vi "RDG822 User.vi"() -> ()   [LabVIEW 2021]
panel:
  in  "MenuCont":u32=1
  in  "RemoveReq?":bool=TRUE
  in  "userID":string="0001"
  out "error out":errorcluster
  in  "E:\\Study\\НИР_Маг\\FP":path=path "E:/Study/НИР_Маг/FP"
  in  "error in":errorcluster
  in  "DutyDBL":dbl=50.0 format="%.3f"
  out "DutyStr":string="50.000 %"
  in  "Noise":bool
  in  "Pulse":bool
  in  "Ramp":bool
  in  "Square":bool
  in  "Sine":bool
  in  "Slider":bool
  in  "PhaseDBL":dbl format="%.3f"
  in  "OK":bool
  out "PhaseStr":string="0.000 °"
  in  "LowL":dbl=-2.5 format="%.4f"
  in  "Offset":dbl format="%.4f"
  out "Offset-LowL":string="0.0000 Vdc"
  in  "Offset/LowL":bool
  in  "HighL":dbl=1.0 format="%.4f"
  in  "Ampl":dbl=5.0 format="%.4f"
  out "Ampl-HighL":string="5.0000 Vpp"
  in  "Ampl/HighL":bool
  in  "Freq":dbl=1.0 format="%.6f"
  in  "Period":dbl=1.0 format="%.7f"
  out "Freq-Period":string="1000.000000000 kHz"
  in  "Freq/Period":bool
  in  "Left":bool
  in  "Right":bool
  in  "Out2":bool
  in  "Out1":bool
  out "Screen":picture
  in  "Menu":bool
  in  "Home":bool
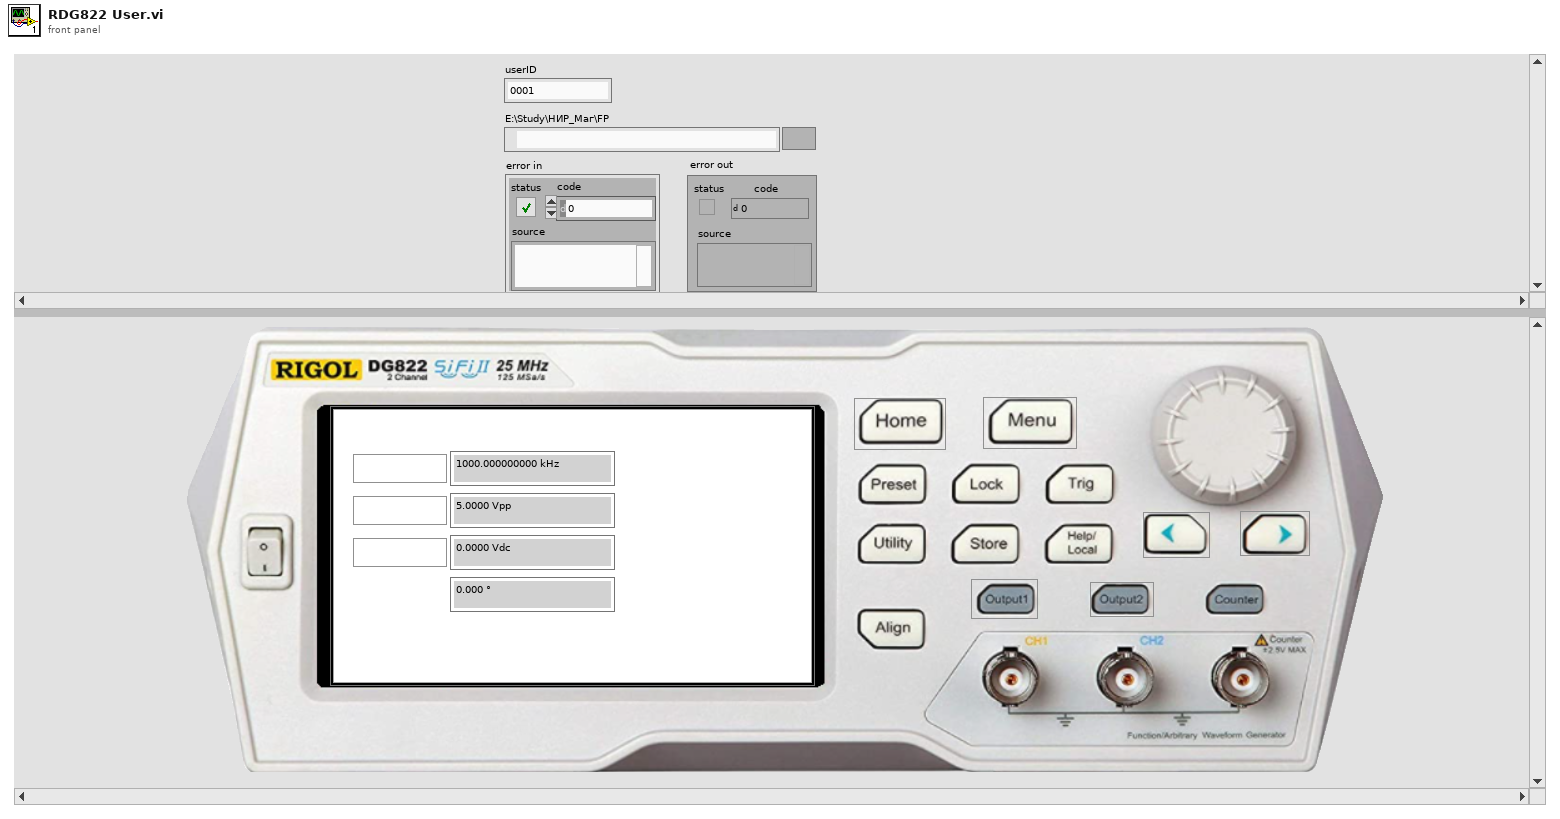
[diagram p1: front panel]
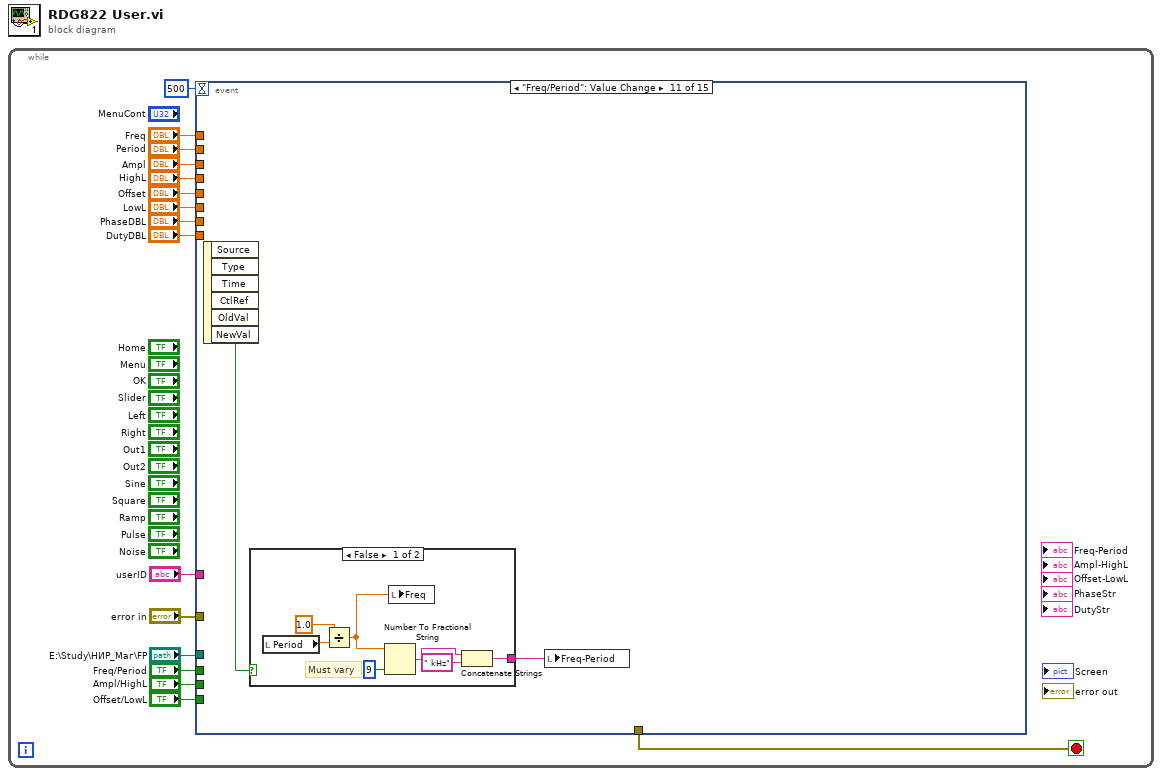
[diagram p0: block diagram]
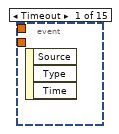
[diagram p2: hidden frame]
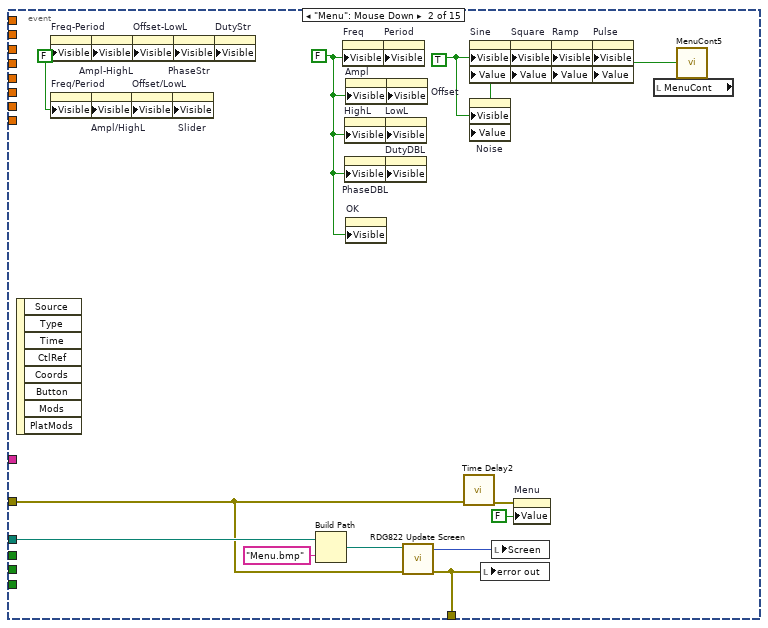
[diagram p3: hidden frame]
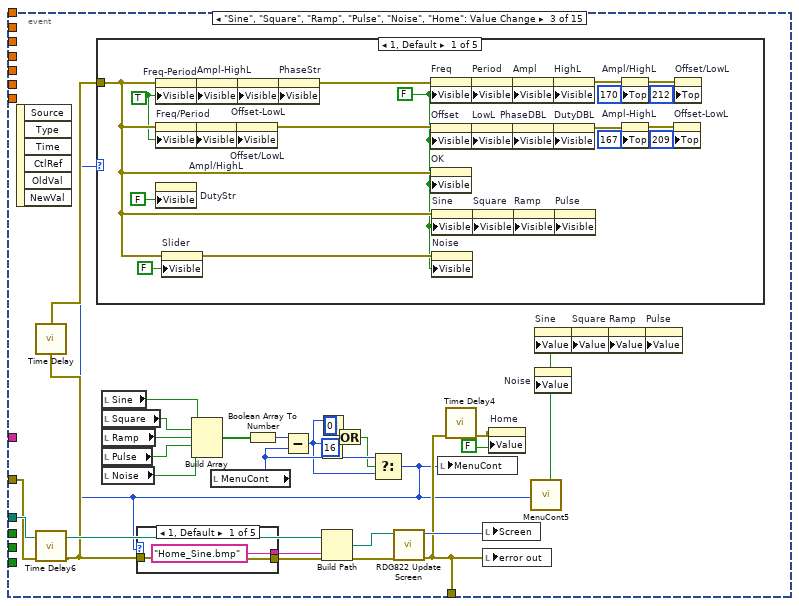
[diagram p4: hidden frame]
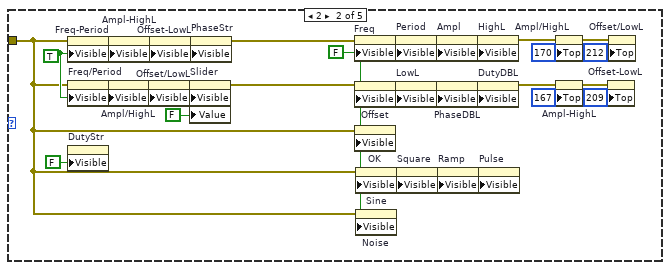
[diagram p5: hidden frame]
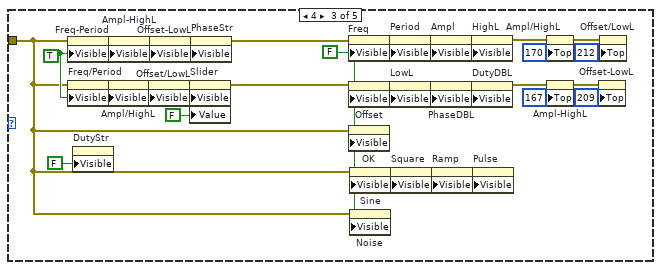
[diagram p6: hidden frame]
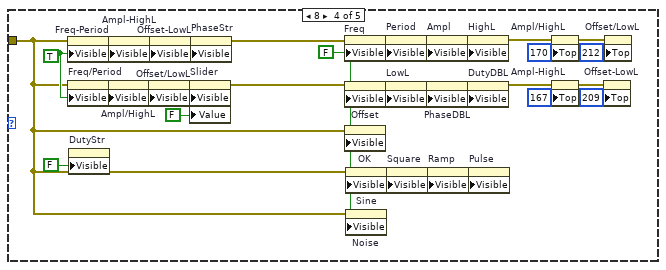
[diagram p7: hidden frame]
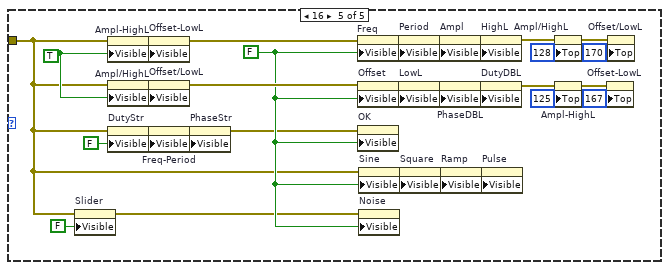
[diagram p8: hidden frame]
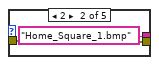
[diagram p9: hidden frame]
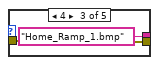
[diagram p10: hidden frame]
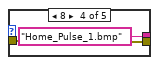
[diagram p11: hidden frame]
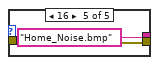
[diagram p12: hidden frame]
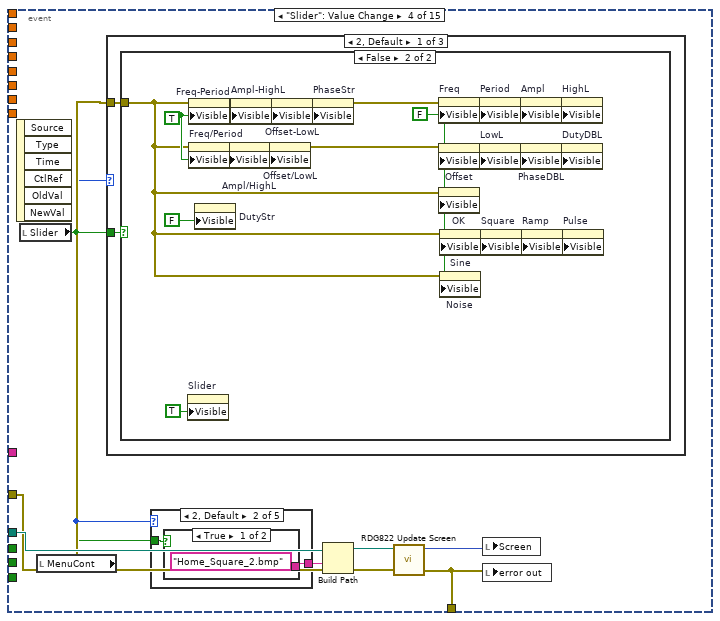
[diagram p13: hidden frame]
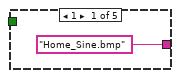
[diagram p14: hidden frame]
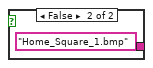
[diagram p15: hidden frame]
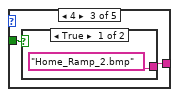
[diagram p16: hidden frame]
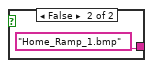
[diagram p17: hidden frame]
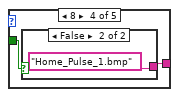
[diagram p18: hidden frame]
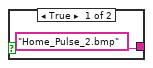
[diagram p19: hidden frame]
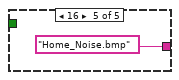
[diagram p20: hidden frame]
diagram:
  n1 = while {
    stop <- w16 stop-if-true
    n2 = event shown="[10] \"Freq/Period\": Value Change" {
      selector: _ -> [_ _ _ _ _ _ _ _ _ _ _ _ _ _ _]
      dyn-events: _ -> [_ _ _ _ _ _ _ _ _ _ _ _ _ _ _]
      timeout: 500 -> [_ _ _ _ _ _ _ _ _ _ _ _ _ _ _]
      tunnel: [_ w39 w64 w236 w393 w770 w803 w836 w868 w889 _ _ _ w1009 _] -> w16
      tunnel: "error in" -> [_ w37 w52 w235 w384 _ _ _ _ _ _ _ _ w1027 _]
      tunnel: "E:\\Study\\НИР_Маг\\FP" -> [_ w40 w68 w237 w397 w785 w818 w851 w874 w895 _ _ _ w1015 _]
      tunnel: "Freq/Period" -> [_ _ _ _ w400 w783 _ _ _ _ _ _ _ w1044 _]
      tunnel: "Ampl/HighL" -> [_ _ _ _ w399 _ w813 _ _ _ _ _ _ w1045 _]
      tunnel: "Freq" -> [_ _ _ _ _ _ _ _ _ _ _ _ _ w1043 _]
      tunnel: "Ampl" -> [_ _ _ _ _ _ _ _ _ _ _ _ _ w1041 _]
      tunnel: "Period" -> [_ _ _ _ _ _ _ _ _ _ _ _ _ w1042 _]
      tunnel: "HighL" -> [_ _ _ _ _ _ _ _ _ _ _ _ _ w1038 _]
      tunnel: "Offset/LowL" -> [_ _ _ _ w398 _ _ w841 _ _ _ _ _ w1040 _]
      tunnel: "Offset" -> [_ _ _ _ _ _ _ _ _ _ _ _ _ w1004 _]
      tunnel: "LowL" -> [_ _ _ _ _ _ _ _ _ _ _ _ _ w1039 _]
      tunnel: "PhaseDBL" -> [_ _ _ _ _ _ _ _ _ _ _ _ _ w1032 _]
      tunnel: "userID" -> [_ _ _ _ _ _ _ _ _ _ _ _ _ w1026 _]
      tunnel: "DutyDBL" -> [_ _ _ _ _ _ _ _ _ _ _ _ _ w1001 _]
      event Timeout {
        n3 = event-data() -> ()  [unwired: 1 in, 3 out]
      }
      event "Menu": Mouse Down {
        w25 = TRUE ("Visible")
        w18 = FALSE ("Visible")
        w17 = FALSE ("Visible")
        n4 = event-data() -> ()  [unwired: 1 in, 8 out]
        n5 = property on="Freq-Period" class="Str"("Visible"=w18) -> (error out=w36:errorcluster)  [unwired: 2 in, 1 out]
        n6 = property on="Freq/Period" class="Bool (strict)"("Visible"=w18) -> (error out=w33:errorcluster)  [unwired: 2 in, 1 out]
        n7 = property on="Ampl/HighL" class="Bool (strict)"(error in=w33, "Visible"=w18) -> (error out=w32:errorcluster)  [unwired: 1 in, 1 out]
        n8 = property on="Ampl-HighL" class="Str"(error in=w36, "Visible"=w18) -> (error out=w35:errorcluster)  [unwired: 1 in, 1 out]
        n9 = property on="Offset/LowL" class="Bool (strict)"(error in=w32, "Visible"=w18) -> (error out=w29:errorcluster)  [unwired: 1 in, 1 out]
        n10 = property on="Offset-LowL" class="Str"(error in=w35, "Visible"=w18) -> (error out=w34:errorcluster)  [unwired: 1 in, 1 out]
        n11 = property on="Slider" class="Bool (strict)"(error in=w29, "Visible"=w18) -> ()  [unwired: 1 in, 2 out]
        n12 = property on="PhaseStr" class="Str"(error in=w34, "Visible"=w18) -> ()  [unwired: 1 in, 2 out]
        n13 = property on="DutyStr" class="Str"("Visible"=w18) -> ()  [unwired: 2 in, 2 out]
        n14 = Build Path(base path=w40, name or relative path="Menu.bmp") -> (appended path=w41:path)
        n15 = property on="Freq" class="DigNum (strict)"("Visible"=w17) -> (error out=w31:errorcluster)  [unwired: 2 in, 1 out]
        n16 = property on="HighL" class="DigNum (strict)"("Visible"=w17) -> ()  [unwired: 2 in, 2 out]
        n17 = property on="PhaseDBL" class="DigNum (strict)"("Visible"=w17) -> ()  [unwired: 2 in, 2 out]
        n18 = property on="Ampl" class="DigNum (strict)"("Visible"=w17) -> (error out=w30:errorcluster)  [unwired: 2 in, 1 out]
        n19 = property on="OK" class="Bool (strict)"("Visible"=w17) -> ()  [unwired: 2 in, 2 out]
        n20 = property on="Period" class="DigNum (strict)"(error in=w31, "Visible"=w17) -> ()  [unwired: 1 in, 2 out]
        n21 = property on="LowL" class="DigNum (strict)"("Visible"=w17) -> ()  [unwired: 2 in, 2 out]
        n22 = property on="DutyDBL" class="DigNum (strict)"("Visible"=w17) -> ()  [unwired: 2 in, 2 out]
        n23 = property on="Offset" class="DigNum (strict)"(error in=w30, "Visible"=w17) -> ()  [unwired: 1 in, 2 out]
        n24 = call "RDG822 Update Screen.vi"("error in"=w37, "Path to file"=w41) -> ("error out"=w39:errorcluster, "Screen"=w38:picture)  [unwired: 8 in]
        n25 = call "Time Delay2"("error in (no error)"=w37) -> ("error out"=w44:errorcluster)  [unwired: 10 in]
        n26 = local write "error out"(w39) -> ()
        n27 = local write "Screen"(w38) -> ()
        n28 = property on="Menu" class="Bool (strict)"(error in=w44, "Value"=FALSE ("Visible")) -> ()  [unwired: 1 in, 2 out]
        n29 = local read "MenuCont"() -> (w24:u32)
        n30 = call "MenuCont5.vi"("MenuID"=w24) -> ("Sine"=w23:bool, "Square"=w22:bool, "Ramp"=w21:bool, "Pulse"=w20:bool, "Noise"=w19:bool)  [unwired: 10 in]
        n31 = property on="Sine" class="Bool (strict)"("Visible"=w25, "Value"=w23) -> (error out=w28:errorcluster)  [unwired: 2 in, 1 out]
        n32 = property on="Noise" class="Bool (strict)"("Visible"=w25, "Value"=w19) -> ()  [unwired: 2 in, 2 out]
        n33 = property on="Square" class="Bool (strict)"(error in=w28, "Visible"=w25, "Value"=w22) -> (error out=w27:errorcluster)  [unwired: 1 in, 1 out]
        n34 = property on="Ramp" class="Bool (strict)"(error in=w27, "Visible"=w25, "Value"=w21) -> (error out=w26:errorcluster)  [unwired: 1 in, 1 out]
        n35 = property on="Pulse" class="Bool (strict)"(error in=w26, "Visible"=w25, "Value"=w20) -> ()  [unwired: 1 in, 2 out]
      }
      event "Sine", "Square", "Ramp", "Pulse", "Noise", "Home": Value Change {
        n36 = event-data() -> ()  [unwired: 1 in, 6 out]
        n37 = call "Time Delay6"("error in (no error)"=w52) -> ("error out"=w49:errorcluster)  [unwired: 10 in]
        n38 = call "Time Delay"("error in (no error)"=w49) -> ("error out"=w50:errorcluster)  [unwired: 10 in]
        n39 = local read "Sine"() -> (w73:bool)
        n40 = local read "Square"() -> (w74:bool)
        n41 = local read "Ramp"() -> (w75:bool)
        n42 = local read "Pulse"() -> (w72:bool)
        n43 = local read "Noise"() -> (w71:bool)
        n44 = Build Array(w73, w74, w75, w72, w71) -> (w76:bool[])
        n45 = local read "MenuCont"() -> (w48:u32)
        n46 = Boolean Array To Number(Boolean array=w76) -> (number=w70:u32)
        n47 = Subtract(x=w70, y=w48) -> (x-y=w47:u32)
        n48 = Greater?(x=w47, y=u32 16) -> (0:w54:bool)
        n49 = Less Or Equal?(x=w47, y=u32 0) -> (x <= y?=w55:bool)
        n50 = Or(x=w55, y=w54) -> (x .or. y?=w46:bool)
        n51 = Select(t=w48, s=w46, f=w47) -> (s? t:f=w45:u32)
        n52 = case shown="1, Default" w45 {
          tunnel: w50 -> [w91 w119 w148 w177 w195]
          frame 1, Default {
            w80 = TRUE ("Visible")
            w81 = FALSE ("Visible")
            n53 = property on="Freq-Period" class="Str"(error in=w91, "Visible"=w80) -> (error out=w107:errorcluster)  [unwired: 1 in, 1 out]
            n54 = property on="Freq/Period" class="Bool (strict)"(error in=w91, "Visible"=w80) -> (error out=w104:errorcluster)  [unwired: 1 in, 1 out]
            n55 = property on="DutyStr" class="Str"("Visible"=FALSE) -> ()  [unwired: 2 in, 2 out]
            n56 = property on="Slider" class="Bool (strict)"(error in=w91, "Visible"=FALSE) -> (error out=w92:errorcluster)  [unwired: 1 in, 1 out]
            n57 = property on="Ampl/HighL" class="Bool (strict)"(error in=w104, "Visible"=w80) -> (error out=w103:errorcluster)  [unwired: 1 in, 1 out]
            n58 = property on="Ampl-HighL" class="Str"(error in=w107, "Visible"=w80) -> (error out=w106:errorcluster)  [unwired: 1 in, 1 out]
            n59 = property on="Offset/LowL" class="Bool (strict)"(error in=w103, "Visible"=w80) -> (error out=w93:errorcluster)  [unwired: 1 in, 1 out]
            n60 = property on="Offset-LowL" class="Str"(error in=w106, "Visible"=w80) -> (error out=w105:errorcluster)  [unwired: 1 in, 1 out]
            n61 = property on="PhaseStr" class="Str"(error in=w105, "Visible"=w80) -> (error out=w98:errorcluster)  [unwired: 1 in, 1 out]
            n62 = property on="Freq" class="DigNum (strict)"(error in=w98, "Visible"=w81) -> (error out=w97:errorcluster)  [unwired: 1 in, 1 out]
            n63 = property on="Offset" class="DigNum (strict)"(error in=w93, "Visible"=w81) -> (error out=w94:errorcluster)  [unwired: 1 in, 1 out]
            n64 = property on="OK" class="Bool (strict)"(error in=w91, "Visible"=w81) -> ()  [unwired: 1 in, 2 out]
            n65 = property on="Sine" class="Bool (strict)"(error in=w91, "Visible"=w81) -> (error out=w101:errorcluster)  [unwired: 1 in, 1 out]
            n66 = property on="Noise" class="Bool (strict)"(error in=w92, "Visible"=w81) -> ()  [unwired: 1 in, 2 out]
            n67 = property on="Period" class="DigNum (strict)"(error in=w97, "Visible"=w81) -> (error out=w96:errorcluster)  [unwired: 1 in, 1 out]
            n68 = property on="LowL" class="DigNum (strict)"(error in=w94, "Visible"=w81) -> (error out=w95:errorcluster)  [unwired: 1 in, 1 out]
            n69 = property on="Square" class="Bool (strict)"(error in=w101, "Visible"=w81) -> (error out=w100:errorcluster)  [unwired: 1 in, 1 out]
            n70 = property on="Ampl" class="DigNum (strict)"(error in=w96, "Visible"=w81) -> (error out=w102:errorcluster)  [unwired: 1 in, 1 out]
            n71 = property on="PhaseDBL" class="DigNum (strict)"(error in=w95, "Visible"=w81) -> (error out=w82:errorcluster)  [unwired: 1 in, 1 out]
            n72 = property on="Ramp" class="Bool (strict)"(error in=w100, "Visible"=w81) -> (error out=w99:errorcluster)  [unwired: 1 in, 1 out]
            n73 = property on="HighL" class="DigNum (strict)"(error in=w102, "Visible"=w81) -> (error out=w88:errorcluster)  [unwired: 1 in, 1 out]
            n74 = property on="DutyDBL" class="DigNum (strict)"("Visible"=w81) -> ()  [unwired: 2 in, 2 out]
            n75 = property on="Pulse" class="Bool (strict)"(error in=w99, "Visible"=w81) -> ()  [unwired: 1 in, 2 out]
            n76 = property on="Ampl/HighL" class="Bool (strict)"(error in=w88, "Top"=170 ("Position:Top")) -> (error out=w86:errorcluster)  [unwired: 1 in, 1 out]
            n77 = property on="Ampl-HighL" class="Str"(error in=w82, "Top"=167 ("Position:Top")) -> (error out=w83:errorcluster)  [unwired: 1 in, 1 out]
            n78 = property on="Offset-LowL" class="Str"(error in=w83, "Top"=209 ("Position:Top")) -> ()  [unwired: 1 in, 2 out]
            n79 = property on="Offset/LowL" class="Bool (strict)"(error in=w86, "Top"=212 ("Position:Top")) -> ()  [unwired: 1 in, 2 out]
          }
          frame 2 {
            w129 = TRUE ("Visible")
            w109 = FALSE ("Visible")
            n80 = property on="Freq-Period" class="Str"(error in=w119, "Visible"=w129) -> (error out=w136:errorcluster)  [unwired: 1 in, 1 out]
            n81 = property on="Freq/Period" class="Bool (strict)"(error in=w119, "Visible"=w129) -> (error out=w133:errorcluster)  [unwired: 1 in, 1 out]
            n82 = property on="DutyStr" class="Str"("Visible"=FALSE) -> ()  [unwired: 2 in, 2 out]
            n83 = property on="Ampl/HighL" class="Bool (strict)"(error in=w133, "Visible"=w129) -> (error out=w132:errorcluster)  [unwired: 1 in, 1 out]
            n84 = property on="Ampl-HighL" class="Str"(error in=w136, "Visible"=w129) -> (error out=w135:errorcluster)  [unwired: 1 in, 1 out]
            n85 = property on="Offset/LowL" class="Bool (strict)"(error in=w132, "Visible"=w129) -> (error out=w130:errorcluster)  [unwired: 1 in, 1 out]
            n86 = property on="Offset-LowL" class="Str"(error in=w135, "Visible"=w129) -> (error out=w134:errorcluster)  [unwired: 1 in, 1 out]
            n87 = property on="Slider" class="Bool (strict)"(error in=w130, "Visible"=w129, "Value"=FALSE ("Slider")) -> (error out=w124:errorcluster)  [unwired: 1 in, 1 out]
            n88 = property on="PhaseStr" class="Str"(error in=w134, "Visible"=w129) -> (error out=w125:errorcluster)  [unwired: 1 in, 1 out]
            n89 = property on="Freq" class="DigNum (strict)"(error in=w125, "Visible"=w109) -> (error out=w123:errorcluster)  [unwired: 1 in, 1 out]
            n90 = property on="Offset" class="DigNum (strict)"(error in=w124, "Visible"=w109) -> (error out=w120:errorcluster)  [unwired: 1 in, 1 out]
            n91 = property on="OK" class="Bool (strict)"(error in=w119, "Visible"=w109) -> ()  [unwired: 1 in, 2 out]
            n92 = property on="Sine" class="Bool (strict)"(error in=w119, "Visible"=w109) -> (error out=w128:errorcluster)  [unwired: 1 in, 1 out]
            n93 = property on="Noise" class="Bool (strict)"(error in=w119, "Visible"=w109) -> ()  [unwired: 1 in, 2 out]
            n94 = property on="Period" class="DigNum (strict)"(error in=w123, "Visible"=w109) -> (error out=w122:errorcluster)  [unwired: 1 in, 1 out]
            n95 = property on="LowL" class="DigNum (strict)"(error in=w120, "Visible"=w109) -> (error out=w121:errorcluster)  [unwired: 1 in, 1 out]
            n96 = property on="Square" class="Bool (strict)"(error in=w128, "Visible"=w109) -> (error out=w127:errorcluster)  [unwired: 1 in, 1 out]
            n97 = property on="Ampl" class="DigNum (strict)"(error in=w122, "Visible"=w109) -> (error out=w131:errorcluster)  [unwired: 1 in, 1 out]
            n98 = property on="PhaseDBL" class="DigNum (strict)"(error in=w121, "Visible"=w109) -> (error out=w111:errorcluster)  [unwired: 1 in, 1 out]
            n99 = property on="Ramp" class="Bool (strict)"(error in=w127, "Visible"=w109) -> (error out=w126:errorcluster)  [unwired: 1 in, 1 out]
            n100 = property on="HighL" class="DigNum (strict)"(error in=w131, "Visible"=w109) -> (error out=w110:errorcluster)  [unwired: 1 in, 1 out]
            n101 = property on="DutyDBL" class="DigNum (strict)"("Visible"=w109) -> ()  [unwired: 2 in, 2 out]
            n102 = property on="Pulse" class="Bool (strict)"(error in=w126, "Visible"=w109) -> ()  [unwired: 1 in, 2 out]
            n103 = property on="Ampl/HighL" class="Bool (strict)"(error in=w110, "Top"=170 ("Position:Top")) -> (error out=w115:errorcluster)  [unwired: 1 in, 1 out]
            n104 = property on="Ampl-HighL" class="Str"(error in=w111, "Top"=167 ("Position:Top")) -> (error out=w112:errorcluster)  [unwired: 1 in, 1 out]
            n105 = property on="Offset-LowL" class="Str"(error in=w112, "Top"=209 ("Position:Top")) -> ()  [unwired: 1 in, 2 out]
            n106 = property on="Offset/LowL" class="Bool (strict)"(error in=w115, "Top"=212 ("Position:Top")) -> ()  [unwired: 1 in, 2 out]
          }
          frame 4 {
            w158 = TRUE ("Visible")
            w138 = FALSE ("Visible")
            n107 = property on="Freq-Period" class="Str"(error in=w148, "Visible"=w158) -> (error out=w165:errorcluster)  [unwired: 1 in, 1 out]
            n108 = property on="Freq/Period" class="Bool (strict)"(error in=w148, "Visible"=w158) -> (error out=w162:errorcluster)  [unwired: 1 in, 1 out]
            n109 = property on="DutyStr" class="Str"("Visible"=FALSE) -> ()  [unwired: 2 in, 2 out]
            n110 = property on="Ampl/HighL" class="Bool (strict)"(error in=w162, "Visible"=w158) -> (error out=w161:errorcluster)  [unwired: 1 in, 1 out]
            n111 = property on="Ampl-HighL" class="Str"(error in=w165, "Visible"=w158) -> (error out=w164:errorcluster)  [unwired: 1 in, 1 out]
            n112 = property on="Offset/LowL" class="Bool (strict)"(error in=w161, "Visible"=w158) -> (error out=w159:errorcluster)  [unwired: 1 in, 1 out]
            n113 = property on="Offset-LowL" class="Str"(error in=w164, "Visible"=w158) -> (error out=w163:errorcluster)  [unwired: 1 in, 1 out]
            n114 = property on="Slider" class="Bool (strict)"(error in=w159, "Visible"=w158, "Value"=FALSE ("Slider")) -> (error out=w153:errorcluster)  [unwired: 1 in, 1 out]
            n115 = property on="PhaseStr" class="Str"(error in=w163, "Visible"=w158) -> (error out=w154:errorcluster)  [unwired: 1 in, 1 out]
            n116 = property on="Freq" class="DigNum (strict)"(error in=w154, "Visible"=w138) -> (error out=w152:errorcluster)  [unwired: 1 in, 1 out]
            n117 = property on="Offset" class="DigNum (strict)"(error in=w153, "Visible"=w138) -> (error out=w149:errorcluster)  [unwired: 1 in, 1 out]
            n118 = property on="OK" class="Bool (strict)"(error in=w148, "Visible"=w138) -> ()  [unwired: 1 in, 2 out]
            n119 = property on="Sine" class="Bool (strict)"(error in=w148, "Visible"=w138) -> (error out=w157:errorcluster)  [unwired: 1 in, 1 out]
            n120 = property on="Noise" class="Bool (strict)"(error in=w148, "Visible"=w138) -> ()  [unwired: 1 in, 2 out]
            n121 = property on="Period" class="DigNum (strict)"(error in=w152, "Visible"=w138) -> (error out=w151:errorcluster)  [unwired: 1 in, 1 out]
            n122 = property on="LowL" class="DigNum (strict)"(error in=w149, "Visible"=w138) -> (error out=w150:errorcluster)  [unwired: 1 in, 1 out]
            n123 = property on="Square" class="Bool (strict)"(error in=w157, "Visible"=w138) -> (error out=w156:errorcluster)  [unwired: 1 in, 1 out]
            n124 = property on="Ampl" class="DigNum (strict)"(error in=w151, "Visible"=w138) -> (error out=w160:errorcluster)  [unwired: 1 in, 1 out]
            n125 = property on="PhaseDBL" class="DigNum (strict)"(error in=w150, "Visible"=w138) -> (error out=w139:errorcluster)  [unwired: 1 in, 1 out]
            n126 = property on="Ramp" class="Bool (strict)"(error in=w156, "Visible"=w138) -> (error out=w155:errorcluster)  [unwired: 1 in, 1 out]
            n127 = property on="HighL" class="DigNum (strict)"(error in=w160, "Visible"=w138) -> (error out=w140:errorcluster)  [unwired: 1 in, 1 out]
            n128 = property on="DutyDBL" class="DigNum (strict)"("Visible"=w138) -> ()  [unwired: 2 in, 2 out]
            n129 = property on="Pulse" class="Bool (strict)"(error in=w155, "Visible"=w138) -> ()  [unwired: 1 in, 2 out]
            n130 = property on="Ampl/HighL" class="Bool (strict)"(error in=w140, "Top"=170 ("Position:Top")) -> (error out=w144:errorcluster)  [unwired: 1 in, 1 out]
            n131 = property on="Ampl-HighL" class="Str"(error in=w139, "Top"=167 ("Position:Top")) -> (error out=w141:errorcluster)  [unwired: 1 in, 1 out]
            n132 = property on="Offset-LowL" class="Str"(error in=w141, "Top"=209 ("Position:Top")) -> ()  [unwired: 1 in, 2 out]
            n133 = property on="Offset/LowL" class="Bool (strict)"(error in=w144, "Top"=212 ("Position:Top")) -> ()  [unwired: 1 in, 2 out]
          }
          frame 8 {
            w187 = TRUE ("Visible")
            w167 = FALSE ("Visible")
            n134 = property on="Freq-Period" class="Str"(error in=w177, "Visible"=w187) -> (error out=w194:errorcluster)  [unwired: 1 in, 1 out]
            n135 = property on="Freq/Period" class="Bool (strict)"(error in=w177, "Visible"=w187) -> (error out=w191:errorcluster)  [unwired: 1 in, 1 out]
            n136 = property on="DutyStr" class="Str"("Visible"=FALSE) -> ()  [unwired: 2 in, 2 out]
            n137 = property on="Ampl/HighL" class="Bool (strict)"(error in=w191, "Visible"=w187) -> (error out=w190:errorcluster)  [unwired: 1 in, 1 out]
            n138 = property on="Ampl-HighL" class="Str"(error in=w194, "Visible"=w187) -> (error out=w193:errorcluster)  [unwired: 1 in, 1 out]
            n139 = property on="Offset/LowL" class="Bool (strict)"(error in=w190, "Visible"=w187) -> (error out=w188:errorcluster)  [unwired: 1 in, 1 out]
            n140 = property on="Offset-LowL" class="Str"(error in=w193, "Visible"=w187) -> (error out=w192:errorcluster)  [unwired: 1 in, 1 out]
            n141 = property on="Slider" class="Bool (strict)"(error in=w188, "Visible"=w187, "Value"=FALSE ("Slider")) -> (error out=w182:errorcluster)  [unwired: 1 in, 1 out]
            n142 = property on="PhaseStr" class="Str"(error in=w192, "Visible"=w187) -> (error out=w183:errorcluster)  [unwired: 1 in, 1 out]
            n143 = property on="Freq" class="DigNum (strict)"(error in=w183, "Visible"=w167) -> (error out=w181:errorcluster)  [unwired: 1 in, 1 out]
            n144 = property on="Offset" class="DigNum (strict)"(error in=w182, "Visible"=w167) -> (error out=w178:errorcluster)  [unwired: 1 in, 1 out]
            n145 = property on="OK" class="Bool (strict)"(error in=w177, "Visible"=w167) -> ()  [unwired: 1 in, 2 out]
            n146 = property on="Sine" class="Bool (strict)"(error in=w177, "Visible"=w167) -> (error out=w186:errorcluster)  [unwired: 1 in, 1 out]
            n147 = property on="Noise" class="Bool (strict)"(error in=w177, "Visible"=w167) -> ()  [unwired: 1 in, 2 out]
            n148 = property on="Period" class="DigNum (strict)"(error in=w181, "Visible"=w167) -> (error out=w180:errorcluster)  [unwired: 1 in, 1 out]
            n149 = property on="LowL" class="DigNum (strict)"(error in=w178, "Visible"=w167) -> (error out=w179:errorcluster)  [unwired: 1 in, 1 out]
            n150 = property on="Square" class="Bool (strict)"(error in=w186, "Visible"=w167) -> (error out=w185:errorcluster)  [unwired: 1 in, 1 out]
            n151 = property on="Ampl" class="DigNum (strict)"(error in=w180, "Visible"=w167) -> (error out=w189:errorcluster)  [unwired: 1 in, 1 out]
            n152 = property on="PhaseDBL" class="DigNum (strict)"(error in=w179, "Visible"=w167) -> (error out=w168:errorcluster)  [unwired: 1 in, 1 out]
            n153 = property on="Ramp" class="Bool (strict)"(error in=w185, "Visible"=w167) -> (error out=w184:errorcluster)  [unwired: 1 in, 1 out]
            n154 = property on="HighL" class="DigNum (strict)"(error in=w189, "Visible"=w167) -> (error out=w169:errorcluster)  [unwired: 1 in, 1 out]
            n155 = property on="DutyDBL" class="DigNum (strict)"("Visible"=w167) -> ()  [unwired: 2 in, 2 out]
            n156 = property on="Pulse" class="Bool (strict)"(error in=w184, "Visible"=w167) -> ()  [unwired: 1 in, 2 out]
            n157 = property on="Ampl/HighL" class="Bool (strict)"(error in=w169, "Top"=170 ("Position:Top")) -> (error out=w173:errorcluster)  [unwired: 1 in, 1 out]
            n158 = property on="Ampl-HighL" class="Str"(error in=w168, "Top"=167 ("Position:Top")) -> (error out=w170:errorcluster)  [unwired: 1 in, 1 out]
            n159 = property on="Offset-LowL" class="Str"(error in=w170, "Top"=209 ("Position:Top")) -> ()  [unwired: 1 in, 2 out]
            n160 = property on="Offset/LowL" class="Bool (strict)"(error in=w173, "Top"=212 ("Position:Top")) -> ()  [unwired: 1 in, 2 out]
          }
          frame 16 {
            w198 = FALSE ("Visible")
            w218 = TRUE ("Visible")
            w199 = FALSE ("Visible")
            n161 = property on="Slider" class="Bool (strict)"(error in=w195, "Visible"=FALSE) -> ()  [unwired: 1 in, 2 out]
            n162 = property on="Ampl-HighL" class="Str"(error in=w195, "Visible"=w218) -> (error out=w221:errorcluster)  [unwired: 1 in, 1 out]
            n163 = property on="Ampl/HighL" class="Bool (strict)"(error in=w195, "Visible"=w218) -> (error out=w220:errorcluster)  [unwired: 1 in, 1 out]
            n164 = property on="DutyStr" class="Str"(error in=w195, "Visible"=w198) -> (error out=w197:errorcluster)  [unwired: 1 in, 1 out]
            n165 = property on="Offset-LowL" class="Str"(error in=w221, "Visible"=w218) -> (error out=w208:errorcluster)  [unwired: 1 in, 1 out]
            n166 = property on="Offset/LowL" class="Bool (strict)"(error in=w220, "Visible"=w218) -> (error out=w210:errorcluster)  [unwired: 1 in, 1 out]
            n167 = property on="Freq-Period" class="Str"(error in=w197, "Visible"=w198) -> (error out=w196:errorcluster)  [unwired: 1 in, 1 out]
            n168 = property on="PhaseStr" class="Str"(error in=w196, "Visible"=w198) -> ()  [unwired: 1 in, 2 out]
            n169 = property on="Freq" class="DigNum (strict)"(error in=w208, "Visible"=w199) -> (error out=w214:errorcluster)  [unwired: 1 in, 1 out]
            n170 = property on="Offset" class="DigNum (strict)"(error in=w210, "Visible"=w199) -> (error out=w211:errorcluster)  [unwired: 1 in, 1 out]
            n171 = property on="OK" class="Bool (strict)"(error in=w195, "Visible"=w199) -> ()  [unwired: 1 in, 2 out]
            n172 = property on="Sine" class="Bool (strict)"(error in=w195, "Visible"=w199) -> (error out=w217:errorcluster)  [unwired: 1 in, 1 out]
            n173 = property on="Noise" class="Bool (strict)"(error in=w195, "Visible"=w199) -> ()  [unwired: 1 in, 2 out]
            n174 = property on="Period" class="DigNum (strict)"(error in=w214, "Visible"=w199) -> (error out=w213:errorcluster)  [unwired: 1 in, 1 out]
            n175 = property on="LowL" class="DigNum (strict)"(error in=w211, "Visible"=w199) -> (error out=w212:errorcluster)  [unwired: 1 in, 1 out]
            n176 = property on="Square" class="Bool (strict)"(error in=w217, "Visible"=w199) -> (error out=w216:errorcluster)  [unwired: 1 in, 1 out]
            n177 = property on="Ampl" class="DigNum (strict)"(error in=w213, "Visible"=w199) -> (error out=w219:errorcluster)  [unwired: 1 in, 1 out]
            n178 = property on="PhaseDBL" class="DigNum (strict)"(error in=w212, "Visible"=w199) -> (error out=w200:errorcluster)  [unwired: 1 in, 1 out]
            n179 = property on="Ramp" class="Bool (strict)"(error in=w216, "Visible"=w199) -> (error out=w215:errorcluster)  [unwired: 1 in, 1 out]
            n180 = property on="HighL" class="DigNum (strict)"(error in=w219, "Visible"=w199) -> (error out=w201:errorcluster)  [unwired: 1 in, 1 out]
            n181 = property on="DutyDBL" class="DigNum (strict)"("Visible"=w199) -> ()  [unwired: 2 in, 2 out]
            n182 = property on="Pulse" class="Bool (strict)"(error in=w215, "Visible"=w199) -> ()  [unwired: 1 in, 2 out]
            n183 = property on="Ampl/HighL" class="Bool (strict)"(error in=w201, "Top"=128 ("Position:Top")) -> (error out=w205:errorcluster)  [unwired: 1 in, 1 out]
            n184 = property on="Ampl-HighL" class="Str"(error in=w200, "Top"=125 ("Position:Top")) -> (error out=w202:errorcluster)  [unwired: 1 in, 1 out]
            n185 = property on="Offset-LowL" class="Str"(error in=w202, "Top"=167 ("Position:Top")) -> ()  [unwired: 1 in, 2 out]
            n186 = property on="Offset/LowL" class="Bool (strict)"(error in=w205, "Top"=170 ("Position:Top")) -> ()  [unwired: 1 in, 2 out]
          }
        }
        n187 = case shown="1, Default" w45 {
          tunnel: ["Home_Sine.bmp" "Home_Square_1.bmp" "Home_Ramp_1.bmp" "Home_Pulse_1.bmp" "Home_Noise.bmp"] -> w69
          tunnel: w49 -> [w222 w224 w226 w228 w230]
          tunnel: [w222 w224 w226 w228 w230] -> w51
          frame 1, Default {
          }
          frame 2 {
          }
          frame 4 {
          }
          frame 8 {
          }
          frame 16 {
          }
        }
        n188 = Build Path(base path=w68, name or relative path=w69) -> (appended path=w78:path)
        n189 = call "RDG822 Update Screen.vi"("error in"=w51, "Path to file"=w78) -> ("error out"=w64:errorcluster, "Screen"=w77:picture)  [unwired: 8 in]
        n190 = local write "MenuCont"(w45) -> ()
        n191 = call "Time Delay4"("error in (no error)"=w64) -> ("error out"=w66:errorcluster)  [unwired: 10 in]
        n192 = local write "Screen"(w77) -> ()
        n193 = local write "error out"(w64) -> ()
        n194 = property on="Home" class="Bool (strict)"(error in=w66, "Value"=FALSE ("Home")) -> ()  [unwired: 1 in, 2 out]
        n195 = call "MenuCont5.vi"("MenuID"=w45) -> ("Sine"=w60:bool, "Square"=w59:bool, "Ramp"=w58:bool, "Pulse"=w57:bool, "Noise"=w56:bool)  [unwired: 10 in]
        n196 = property on="Sine" class="Bool (strict)"("Value"=w60) -> (error out=w63:errorcluster)  [unwired: 2 in, 1 out]
        n197 = property on="Noise" class="Bool (strict)"("Value"=w56) -> ()  [unwired: 2 in, 2 out]
        n198 = property on="Square" class="Bool (strict)"(error in=w63, "Value"=w59) -> (error out=w62:errorcluster)  [unwired: 1 in, 1 out]
        n199 = property on="Ramp" class="Bool (strict)"(error in=w62, "Value"=w58) -> (error out=w61:errorcluster)  [unwired: 1 in, 1 out]
        n200 = property on="Pulse" class="Bool (strict)"(error in=w61, "Value"=w57) -> ()  [unwired: 1 in, 2 out]
      }
      event "Slider": Value Change {
        n201 = event-data() -> ()  [unwired: 1 in, 6 out]
        n202 = local read "Slider"() -> (w233:bool)
        n203 = local read "MenuCont"() -> (w234:u32)
        n204 = case shown="2, Default" w234 {
          tunnel: w235 -> [w255 w297 w340]
          tunnel: w233 -> [w254 w296 w339]
          frame 2, Default {
            n205 = case shown="False" w254 {
              tunnel: w255 -> [w260 w280]
              frame True {
                w269 = FALSE ("Visible")
                w256 = FALSE ("Visible")
                n206 = property on="Slider" class="Bool (strict)"("Visible"=TRUE) -> ()  [unwired: 2 in, 2 out]
                n207 = property on="Freq-Period" class="Str"(error in=w260, "Visible"=w269) -> (error out=w275:errorcluster)  [unwired: 1 in, 1 out]
                n208 = property on="Freq/Period" class="Bool (strict)"(error in=w260, "Visible"=w269) -> (error out=w272:errorcluster)  [unwired: 1 in, 1 out]
                n209 = property on="DutyStr" class="Str"("Visible"=TRUE) -> ()  [unwired: 2 in, 2 out]
                n210 = property on="Ampl/HighL" class="Bool (strict)"(error in=w272, "Visible"=w269) -> (error out=w271:errorcluster)  [unwired: 1 in, 1 out]
                n211 = property on="Ampl-HighL" class="Str"(error in=w275, "Visible"=w269) -> (error out=w274:errorcluster)  [unwired: 1 in, 1 out]
                n212 = property on="Offset/LowL" class="Bool (strict)"(error in=w271, "Visible"=w269) -> (error out=w259:errorcluster)  [unwired: 1 in, 1 out]
                n213 = property on="Offset-LowL" class="Str"(error in=w274, "Visible"=w269) -> (error out=w273:errorcluster)  [unwired: 1 in, 1 out]
                n214 = property on="PhaseStr" class="Str"(error in=w273, "Visible"=w269) -> (error out=w265:errorcluster)  [unwired: 1 in, 1 out]
                n215 = property on="Freq" class="DigNum (strict)"(error in=w265, "Visible"=w256) -> (error out=w264:errorcluster)  [unwired: 1 in, 1 out]
                n216 = property on="Offset" class="DigNum (strict)"(error in=w259, "Visible"=w256) -> (error out=w261:errorcluster)  [unwired: 1 in, 1 out]
                n217 = property on="OK" class="Bool (strict)"(error in=w260, "Visible"=w256) -> ()  [unwired: 1 in, 2 out]
                n218 = property on="Sine" class="Bool (strict)"(error in=w260, "Visible"=w256) -> (error out=w268:errorcluster)  [unwired: 1 in, 1 out]
                n219 = property on="Noise" class="Bool (strict)"(error in=w260, "Visible"=w256) -> ()  [unwired: 1 in, 2 out]
                n220 = property on="Period" class="DigNum (strict)"(error in=w264, "Visible"=w256) -> (error out=w263:errorcluster)  [unwired: 1 in, 1 out]
                n221 = property on="LowL" class="DigNum (strict)"(error in=w261, "Visible"=w256) -> (error out=w262:errorcluster)  [unwired: 1 in, 1 out]
                n222 = property on="Square" class="Bool (strict)"(error in=w268, "Visible"=w256) -> (error out=w267:errorcluster)  [unwired: 1 in, 1 out]
                n223 = property on="Ampl" class="DigNum (strict)"(error in=w263, "Visible"=w256) -> (error out=w270:errorcluster)  [unwired: 1 in, 1 out]
                n224 = property on="PhaseDBL" class="DigNum (strict)"(error in=w262, "Visible"=w256) -> ()  [unwired: 1 in, 2 out]
                n225 = property on="Ramp" class="Bool (strict)"(error in=w267, "Visible"=w256) -> (error out=w266:errorcluster)  [unwired: 1 in, 1 out]
                n226 = property on="HighL" class="DigNum (strict)"(error in=w270, "Visible"=w256) -> ()  [unwired: 1 in, 2 out]
                n227 = property on="DutyDBL" class="DigNum (strict)"("Visible"=w256) -> ()  [unwired: 2 in, 2 out]
                n228 = property on="Pulse" class="Bool (strict)"(error in=w266, "Visible"=w256) -> ()  [unwired: 1 in, 2 out]
              }
              frame False {
                w289 = TRUE ("Visible")
                w276 = FALSE ("Visible")
                n229 = property on="Slider" class="Bool (strict)"("Visible"=TRUE) -> ()  [unwired: 2 in, 2 out]
                n230 = property on="Freq-Period" class="Str"(error in=w280, "Visible"=w289) -> (error out=w295:errorcluster)  [unwired: 1 in, 1 out]
                n231 = property on="Freq/Period" class="Bool (strict)"(error in=w280, "Visible"=w289) -> (error out=w292:errorcluster)  [unwired: 1 in, 1 out]
                n232 = property on="DutyStr" class="Str"("Visible"=FALSE) -> ()  [unwired: 2 in, 2 out]
                n233 = property on="Ampl/HighL" class="Bool (strict)"(error in=w292, "Visible"=w289) -> (error out=w291:errorcluster)  [unwired: 1 in, 1 out]
                n234 = property on="Ampl-HighL" class="Str"(error in=w295, "Visible"=w289) -> (error out=w294:errorcluster)  [unwired: 1 in, 1 out]
                n235 = property on="Offset/LowL" class="Bool (strict)"(error in=w291, "Visible"=w289) -> (error out=w279:errorcluster)  [unwired: 1 in, 1 out]
                n236 = property on="Offset-LowL" class="Str"(error in=w294, "Visible"=w289) -> (error out=w293:errorcluster)  [unwired: 1 in, 1 out]
                n237 = property on="PhaseStr" class="Str"(error in=w293, "Visible"=w289) -> (error out=w285:errorcluster)  [unwired: 1 in, 1 out]
                n238 = property on="Freq" class="DigNum (strict)"(error in=w285, "Visible"=w276) -> (error out=w284:errorcluster)  [unwired: 1 in, 1 out]
                n239 = property on="Offset" class="DigNum (strict)"(error in=w279, "Visible"=w276) -> (error out=w281:errorcluster)  [unwired: 1 in, 1 out]
                n240 = property on="OK" class="Bool (strict)"(error in=w280, "Visible"=w276) -> ()  [unwired: 1 in, 2 out]
                n241 = property on="Sine" class="Bool (strict)"(error in=w280, "Visible"=w276) -> (error out=w288:errorcluster)  [unwired: 1 in, 1 out]
                n242 = property on="Noise" class="Bool (strict)"(error in=w280, "Visible"=w276) -> ()  [unwired: 1 in, 2 out]
                n243 = property on="Period" class="DigNum (strict)"(error in=w284, "Visible"=w276) -> (error out=w283:errorcluster)  [unwired: 1 in, 1 out]
                n244 = property on="LowL" class="DigNum (strict)"(error in=w281, "Visible"=w276) -> (error out=w282:errorcluster)  [unwired: 1 in, 1 out]
                n245 = property on="Square" class="Bool (strict)"(error in=w288, "Visible"=w276) -> (error out=w287:errorcluster)  [unwired: 1 in, 1 out]
                n246 = property on="Ampl" class="DigNum (strict)"(error in=w283, "Visible"=w276) -> (error out=w290:errorcluster)  [unwired: 1 in, 1 out]
                n247 = property on="PhaseDBL" class="DigNum (strict)"(error in=w282, "Visible"=w276) -> ()  [unwired: 1 in, 2 out]
                n248 = property on="Ramp" class="Bool (strict)"(error in=w287, "Visible"=w276) -> (error out=w286:errorcluster)  [unwired: 1 in, 1 out]
                n249 = property on="HighL" class="DigNum (strict)"(error in=w290, "Visible"=w276) -> ()  [unwired: 1 in, 2 out]
                n250 = property on="DutyDBL" class="DigNum (strict)"("Visible"=w276) -> ()  [unwired: 2 in, 2 out]
                n251 = property on="Pulse" class="Bool (strict)"(error in=w286, "Visible"=w276) -> ()  [unwired: 1 in, 2 out]
              }
            }
          }
          frame 4 {
            n252 = case shown="True" w296 {
              tunnel: w297 -> [w303 w323]
              frame True {
                w311 = FALSE ("Visible")
                w298 = FALSE ("Visible")
                n253 = property on="Freq-Period" class="Str"(error in=w303, "Visible"=w311) -> (error out=w317:errorcluster)  [unwired: 1 in, 1 out]
                n254 = property on="Freq/Period" class="Bool (strict)"(error in=w303, "Visible"=w311) -> (error out=w314:errorcluster)  [unwired: 1 in, 1 out]
                n255 = property on="DutyStr" class="Str"("Visible"=FALSE) -> ()  [unwired: 2 in, 2 out]
                n256 = property on="Slider" class="Bool (strict)"("Visible"=TRUE) -> ()  [unwired: 2 in, 2 out]
                n257 = property on="Ampl/HighL" class="Bool (strict)"(error in=w314, "Visible"=w311) -> (error out=w313:errorcluster)  [unwired: 1 in, 1 out]
                n258 = property on="Ampl-HighL" class="Str"(error in=w317, "Visible"=w311) -> (error out=w316:errorcluster)  [unwired: 1 in, 1 out]
                n259 = property on="Offset/LowL" class="Bool (strict)"(error in=w313, "Visible"=w311) -> (error out=w302:errorcluster)  [unwired: 1 in, 1 out]
                n260 = property on="Offset-LowL" class="Str"(error in=w316, "Visible"=w311) -> (error out=w315:errorcluster)  [unwired: 1 in, 1 out]
                n261 = property on="PhaseStr" class="Str"(error in=w315, "Visible"=w311) -> (error out=w307:errorcluster)  [unwired: 1 in, 1 out]
                n262 = property on="Freq" class="DigNum (strict)"(error in=w307, "Visible"=w298) -> (error out=w306:errorcluster)  [unwired: 1 in, 1 out]
                n263 = property on="Offset" class="DigNum (strict)"(error in=w302, "Visible"=w298) -> (error out=w304:errorcluster)  [unwired: 1 in, 1 out]
                n264 = property on="OK" class="Bool (strict)"(error in=w303, "Visible"=w298) -> ()  [unwired: 1 in, 2 out]
                n265 = property on="Sine" class="Bool (strict)"(error in=w303, "Visible"=w298) -> (error out=w310:errorcluster)  [unwired: 1 in, 1 out]
                n266 = property on="Noise" class="Bool (strict)"(error in=w303, "Visible"=w298) -> ()  [unwired: 1 in, 2 out]
                n267 = property on="Period" class="DigNum (strict)"(error in=w306, "Visible"=w298) -> (error out=w305:errorcluster)  [unwired: 1 in, 1 out]
                n268 = property on="LowL" class="DigNum (strict)"(error in=w304, "Visible"=w298) -> (error out=w299:errorcluster)  [unwired: 1 in, 1 out]
                n269 = property on="Square" class="Bool (strict)"(error in=w310, "Visible"=w298) -> (error out=w309:errorcluster)  [unwired: 1 in, 1 out]
                n270 = property on="Ampl" class="DigNum (strict)"(error in=w305, "Visible"=w298) -> (error out=w312:errorcluster)  [unwired: 1 in, 1 out]
                n271 = property on="PhaseDBL" class="DigNum (strict)"(error in=w299, "Visible"=w298) -> ()  [unwired: 1 in, 2 out]
                n272 = property on="Ramp" class="Bool (strict)"(error in=w309, "Visible"=w298) -> (error out=w308:errorcluster)  [unwired: 1 in, 1 out]
                n273 = property on="HighL" class="DigNum (strict)"(error in=w312, "Visible"=w298) -> ()  [unwired: 1 in, 2 out]
                n274 = property on="DutyDBL" class="DigNum (strict)"(error in=w299, "Visible"=w298) -> ()  [unwired: 1 in, 2 out]
                n275 = property on="Pulse" class="Bool (strict)"(error in=w308, "Visible"=w298) -> ()  [unwired: 1 in, 2 out]
              }
              frame False {
                w332 = TRUE ("Visible")
                w319 = FALSE ("Visible")
                n276 = property on="Freq-Period" class="Str"(error in=w323, "Visible"=w332) -> (error out=w338:errorcluster)  [unwired: 1 in, 1 out]
                n277 = property on="Freq/Period" class="Bool (strict)"(error in=w323, "Visible"=w332) -> (error out=w335:errorcluster)  [unwired: 1 in, 1 out]
                n278 = property on="DutyStr" class="Str"("Visible"=FALSE) -> ()  [unwired: 2 in, 2 out]
                n279 = property on="Slider" class="Bool (strict)"("Visible"=TRUE) -> ()  [unwired: 2 in, 2 out]
                n280 = property on="Ampl/HighL" class="Bool (strict)"(error in=w335, "Visible"=w332) -> (error out=w334:errorcluster)  [unwired: 1 in, 1 out]
                n281 = property on="Ampl-HighL" class="Str"(error in=w338, "Visible"=w332) -> (error out=w337:errorcluster)  [unwired: 1 in, 1 out]
                n282 = property on="Offset/LowL" class="Bool (strict)"(error in=w334, "Visible"=w332) -> (error out=w322:errorcluster)  [unwired: 1 in, 1 out]
                n283 = property on="Offset-LowL" class="Str"(error in=w337, "Visible"=w332) -> (error out=w336:errorcluster)  [unwired: 1 in, 1 out]
                n284 = property on="PhaseStr" class="Str"(error in=w336, "Visible"=w332) -> (error out=w328:errorcluster)  [unwired: 1 in, 1 out]
                n285 = property on="Freq" class="DigNum (strict)"(error in=w328, "Visible"=w319) -> (error out=w327:errorcluster)  [unwired: 1 in, 1 out]
                n286 = property on="Offset" class="DigNum (strict)"(error in=w322, "Visible"=w319) -> (error out=w324:errorcluster)  [unwired: 1 in, 1 out]
                n287 = property on="OK" class="Bool (strict)"(error in=w323, "Visible"=w319) -> ()  [unwired: 1 in, 2 out]
                n288 = property on="Sine" class="Bool (strict)"(error in=w323, "Visible"=w319) -> (error out=w331:errorcluster)  [unwired: 1 in, 1 out]
                n289 = property on="Noise" class="Bool (strict)"(error in=w323, "Visible"=w319) -> ()  [unwired: 1 in, 2 out]
                n290 = property on="Period" class="DigNum (strict)"(error in=w327, "Visible"=w319) -> (error out=w326:errorcluster)  [unwired: 1 in, 1 out]
                n291 = property on="LowL" class="DigNum (strict)"(error in=w324, "Visible"=w319) -> (error out=w325:errorcluster)  [unwired: 1 in, 1 out]
                n292 = property on="Square" class="Bool (strict)"(error in=w331, "Visible"=w319) -> (error out=w330:errorcluster)  [unwired: 1 in, 1 out]
                n293 = property on="Ampl" class="DigNum (strict)"(error in=w326, "Visible"=w319) -> (error out=w333:errorcluster)  [unwired: 1 in, 1 out]
                n294 = property on="PhaseDBL" class="DigNum (strict)"(error in=w325, "Visible"=w319) -> (error out=w320:errorcluster)  [unwired: 1 in, 1 out]
                n295 = property on="Ramp" class="Bool (strict)"(error in=w330, "Visible"=w319) -> (error out=w329:errorcluster)  [unwired: 1 in, 1 out]
                n296 = property on="HighL" class="DigNum (strict)"(error in=w333, "Visible"=w319) -> ()  [unwired: 1 in, 2 out]
                n297 = property on="DutyDBL" class="DigNum (strict)"(error in=w320, "Visible"=w319) -> ()  [unwired: 1 in, 2 out]
                n298 = property on="Pulse" class="Bool (strict)"(error in=w329, "Visible"=w319) -> ()  [unwired: 1 in, 2 out]
              }
            }
          }
          frame 8 {
            n299 = case shown="False" w339 {
              tunnel: w340 -> [w346 w367]
              frame True {
                w355 = FALSE ("Visible")
                w342 = FALSE ("Visible")
                n300 = property on="Freq-Period" class="Str"(error in=w346, "Visible"=w355) -> (error out=w361:errorcluster)  [unwired: 1 in, 1 out]
                n301 = property on="Freq/Period" class="Bool (strict)"(error in=w346, "Visible"=w355) -> (error out=w358:errorcluster)  [unwired: 1 in, 1 out]
                n302 = property on="DutyStr" class="Str"("Visible"=TRUE) -> ()  [unwired: 2 in, 2 out]
                n303 = property on="Slider" class="Bool (strict)"("Visible"=TRUE) -> ()  [unwired: 2 in, 2 out]
                n304 = property on="Ampl/HighL" class="Bool (strict)"(error in=w358, "Visible"=w355) -> (error out=w357:errorcluster)  [unwired: 1 in, 1 out]
                n305 = property on="Ampl-HighL" class="Str"(error in=w361, "Visible"=w355) -> (error out=w360:errorcluster)  [unwired: 1 in, 1 out]
                n306 = property on="Offset/LowL" class="Bool (strict)"(error in=w357, "Visible"=w355) -> (error out=w345:errorcluster)  [unwired: 1 in, 1 out]
                n307 = property on="Offset-LowL" class="Str"(error in=w360, "Visible"=w355) -> (error out=w359:errorcluster)  [unwired: 1 in, 1 out]
                n308 = property on="PhaseStr" class="Str"(error in=w359, "Visible"=w355) -> (error out=w351:errorcluster)  [unwired: 1 in, 1 out]
                n309 = property on="Freq" class="DigNum (strict)"(error in=w351, "Visible"=w342) -> (error out=w350:errorcluster)  [unwired: 1 in, 1 out]
                n310 = property on="Offset" class="DigNum (strict)"(error in=w345, "Visible"=w342) -> (error out=w347:errorcluster)  [unwired: 1 in, 1 out]
                n311 = property on="OK" class="Bool (strict)"(error in=w346, "Visible"=w342) -> ()  [unwired: 1 in, 2 out]
                n312 = property on="Sine" class="Bool (strict)"(error in=w346, "Visible"=w342) -> (error out=w354:errorcluster)  [unwired: 1 in, 1 out]
                n313 = property on="Noise" class="Bool (strict)"(error in=w346, "Visible"=w342) -> ()  [unwired: 1 in, 2 out]
                n314 = property on="Period" class="DigNum (strict)"(error in=w350, "Visible"=w342) -> (error out=w349:errorcluster)  [unwired: 1 in, 1 out]
                n315 = property on="LowL" class="DigNum (strict)"(error in=w347, "Visible"=w342) -> (error out=w348:errorcluster)  [unwired: 1 in, 1 out]
                n316 = property on="Square" class="Bool (strict)"(error in=w354, "Visible"=w342) -> (error out=w353:errorcluster)  [unwired: 1 in, 1 out]
                n317 = property on="Ampl" class="DigNum (strict)"(error in=w349, "Visible"=w342) -> (error out=w356:errorcluster)  [unwired: 1 in, 1 out]
                n318 = property on="PhaseDBL" class="DigNum (strict)"(error in=w348, "Visible"=w342) -> (error out=w341:errorcluster)  [unwired: 1 in, 1 out]
                n319 = property on="Ramp" class="Bool (strict)"(error in=w353, "Visible"=w342) -> (error out=w352:errorcluster)  [unwired: 1 in, 1 out]
                n320 = property on="HighL" class="DigNum (strict)"(error in=w356, "Visible"=w342) -> ()  [unwired: 1 in, 2 out]
                n321 = property on="DutyDBL" class="DigNum (strict)"(error in=w341, "Visible"=w342) -> ()  [unwired: 1 in, 2 out]
                n322 = property on="Pulse" class="Bool (strict)"(error in=w352, "Visible"=w342) -> ()  [unwired: 1 in, 2 out]
              }
              frame False {
                w375 = TRUE ("Visible")
                w363 = FALSE ("Visible")
                n323 = property on="Freq-Period" class="Str"(error in=w367, "Visible"=w375) -> (error out=w381:errorcluster)  [unwired: 1 in, 1 out]
                n324 = property on="Freq/Period" class="Bool (strict)"(error in=w367, "Visible"=w375) -> (error out=w378:errorcluster)  [unwired: 1 in, 1 out]
                n325 = property on="DutyStr" class="Str"("Visible"=FALSE) -> ()  [unwired: 2 in, 2 out]
                n326 = property on="Slider" class="Bool (strict)"("Visible"=TRUE) -> ()  [unwired: 2 in, 2 out]
                n327 = property on="Ampl/HighL" class="Bool (strict)"(error in=w378, "Visible"=w375) -> (error out=w377:errorcluster)  [unwired: 1 in, 1 out]
                n328 = property on="Ampl-HighL" class="Str"(error in=w381, "Visible"=w375) -> (error out=w380:errorcluster)  [unwired: 1 in, 1 out]
                n329 = property on="Offset/LowL" class="Bool (strict)"(error in=w377, "Visible"=w375) -> (error out=w366:errorcluster)  [unwired: 1 in, 1 out]
                n330 = property on="Offset-LowL" class="Str"(error in=w380, "Visible"=w375) -> (error out=w379:errorcluster)  [unwired: 1 in, 1 out]
                n331 = property on="PhaseStr" class="Str"(error in=w379, "Visible"=w375) -> (error out=w371:errorcluster)  [unwired: 1 in, 1 out]
                n332 = property on="Freq" class="DigNum (strict)"(error in=w371, "Visible"=w363) -> (error out=w370:errorcluster)  [unwired: 1 in, 1 out]
                n333 = property on="Offset" class="DigNum (strict)"(error in=w366, "Visible"=w363) -> (error out=w368:errorcluster)  [unwired: 1 in, 1 out]
                n334 = property on="OK" class="Bool (strict)"(error in=w367, "Visible"=w363) -> ()  [unwired: 1 in, 2 out]
                n335 = property on="Sine" class="Bool (strict)"(error in=w367, "Visible"=w363) -> (error out=w374:errorcluster)  [unwired: 1 in, 1 out]
                n336 = property on="Noise" class="Bool (strict)"(error in=w367, "Visible"=w363) -> ()  [unwired: 1 in, 2 out]
                n337 = property on="Period" class="DigNum (strict)"(error in=w370, "Visible"=w363) -> (error out=w369:errorcluster)  [unwired: 1 in, 1 out]
                n338 = property on="LowL" class="DigNum (strict)"(error in=w368, "Visible"=w363) -> (error out=w362:errorcluster)  [unwired: 1 in, 1 out]
                n339 = property on="Square" class="Bool (strict)"(error in=w374, "Visible"=w363) -> (error out=w373:errorcluster)  [unwired: 1 in, 1 out]
                n340 = property on="Ampl" class="DigNum (strict)"(error in=w369, "Visible"=w363) -> (error out=w376:errorcluster)  [unwired: 1 in, 1 out]
                n341 = property on="PhaseDBL" class="DigNum (strict)"(error in=w362, "Visible"=w363) -> ()  [unwired: 1 in, 2 out]
                n342 = property on="Ramp" class="Bool (strict)"(error in=w373, "Visible"=w363) -> (error out=w372:errorcluster)  [unwired: 1 in, 1 out]
                n343 = property on="HighL" class="DigNum (strict)"(error in=w376, "Visible"=w363) -> ()  [unwired: 1 in, 2 out]
                n344 = property on="DutyDBL" class="DigNum (strict)"(error in=w362, "Visible"=w363) -> ()  [unwired: 1 in, 2 out]
                n345 = property on="Pulse" class="Bool (strict)"(error in=w372, "Visible"=w363) -> ()  [unwired: 1 in, 2 out]
              }
            }
          }
        }
        n346 = case shown="2, Default" w234 {
          tunnel: ["Home_Sine.bmp" w242 w246 w250 "Home_Noise.bmp"] -> w232
          tunnel: w233 -> [_ w241 w245 w249 _]
          frame 1 {
          }
          frame 2, Default {
            n347 = case shown="True" w241 {
              tunnel: ["Home_Square_2.bmp" "Home_Square_1.bmp"] -> w242
              frame True {
              }
              frame False {
              }
            }
          }
          frame 4 {
            n348 = case shown="True" w245 {
              tunnel: ["Home_Ramp_2.bmp" "Home_Ramp_1.bmp"] -> w246
              frame True {
              }
              frame False {
              }
            }
          }
          frame 8 {
            n349 = case shown="False" w249 {
              tunnel: ["Home_Pulse_2.bmp" "Home_Pulse_1.bmp"] -> w250
              frame True {
              }
              frame False {
              }
            }
          }
          frame 16 {
          }
        }
        n350 = Build Path(base path=w237, name or relative path=w232) -> (appended path=w239:path)
        n351 = call "RDG822 Update Screen.vi"("error in"=w235, "Path to file"=w239) -> ("error out"=w236:errorcluster, "Screen"=w238:picture)  [unwired: 8 in]
        n352 = local write "Screen"(w238) -> ()
        n353 = local write "error out"(w236) -> ()
      }
      event "OK": Mouse Down {
        # "Сделать пересчет"
        n354 = event-data() -> ()  [unwired: 1 in, 8 out]
        n355 = local read "MenuCont"() -> (w382:u32)
        n356 = local read "Slider"() -> (w387:bool)
        n357 = call "Time Delay7"("error in (no error)"=w384) -> ("error out"=w383:errorcluster)  [unwired: 10 in]
        n358 = case shown="1, Default" w382 {
          tunnel: w387 -> [_ w422 w472 w523 _]
          tunnel: w383 -> [w403 w421 w471 w522 w576]
          tunnel: ["Home_Sine.bmp" w420 w470 w521 "Home_Noise.bmp"] -> w386
          tunnel: [w402 w419 w469 w520 w578] -> w385
          frame 1, Default {
            w418 = FALSE ("Visible")
            w407 = TRUE ("Visible")
            n359 = property on="Freq-Period" class="Str"(error in=w403, "Visible"=w407) -> (error out=w412:errorcluster)  [unwired: 1 in, 1 out]
            n360 = property on="Freq/Period" class="Bool (strict)"(error in=w403, "Visible"=w407) -> (error out=w409:errorcluster)  [unwired: 1 in, 1 out]
            n361 = property on="DutyStr" class="Str"(error in=w403, "Visible"=FALSE) -> ()  [unwired: 1 in, 2 out]
            n362 = property on="Slider" class="Bool (strict)"(error in=w403, "Visible"=FALSE) -> ()  [unwired: 1 in, 2 out]
            n363 = property on="Ampl/HighL" class="Bool (strict)"(error in=w409, "Visible"=w407) -> (error out=w408:errorcluster)  [unwired: 1 in, 1 out]
            n364 = property on="Ampl-HighL" class="Str"(error in=w412, "Visible"=w407) -> (error out=w411:errorcluster)  [unwired: 1 in, 1 out]
            n365 = property on="Offset/LowL" class="Bool (strict)"(error in=w408, "Visible"=w407) -> ()  [unwired: 1 in, 2 out]
            n366 = property on="Offset-LowL" class="Str"(error in=w411, "Visible"=w407) -> (error out=w410:errorcluster)  [unwired: 1 in, 1 out]
            n367 = property on="PhaseStr" class="Str"(error in=w410, "Visible"=w407) -> (error out=w417:errorcluster)  [unwired: 1 in, 1 out]
            n368 = property on="Freq" class="DigNum (strict)"(error in=w417, "Visible"=w418) -> (error out=w416:errorcluster)  [unwired: 1 in, 1 out]
            n369 = property on="OK" class="Bool (strict)"("Visible"=w418) -> (error out=w401:errorcluster)  [unwired: 2 in, 1 out]
            n370 = property on="DutyDBL" class="DigNum (strict)"("Visible"=w418) -> ()  [unwired: 2 in, 2 out]
            n371 = property on="Period" class="DigNum (strict)"(error in=w416, "Visible"=w418) -> (error out=w413:errorcluster)  [unwired: 1 in, 1 out]
            n372 = property on="Offset" class="DigNum (strict)"(error in=w413, "Visible"=w418) -> (error out=w414:errorcluster)  [unwired: 1 in, 1 out]
            n373 = property on="PhaseDBL" class="DigNum (strict)"(error in=w413, "Visible"=w418) -> ()  [unwired: 1 in, 2 out]
            n374 = property on="Ampl" class="DigNum (strict)"(error in=w413, "Visible"=w418) -> (error out=w415:errorcluster)  [unwired: 1 in, 1 out]
            n375 = property on="LowL" class="DigNum (strict)"(error in=w414, "Visible"=w418) -> ()  [unwired: 1 in, 2 out]
            n376 = property on="HighL" class="DigNum (strict)"(error in=w415, "Visible"=w418) -> ()  [unwired: 1 in, 2 out]
            n377 = property on="OK" class="Bool (strict)"(error in=w401, "Value"=w418) -> (error out=w402:errorcluster)  [unwired: 1 in, 1 out]
          }
          frame 2 {
            n378 = case shown="True" w422 {
              tunnel: w421 -> [w430 w453]
              tunnel: ["Home_Square_2.bmp" "Home_Square_1.bmp"] -> w420
              tunnel: [w424 w447] -> w419
              frame True {
                w439 = FALSE ("Visible")
                w425 = FALSE ("Visible")
                n379 = property on="Slider" class="Bool (strict)"("Visible"=TRUE) -> ()  [unwired: 2 in, 2 out]
                n380 = property on="Freq-Period" class="Str"(error in=w430, "Visible"=w439) -> (error out=w445:errorcluster)  [unwired: 1 in, 1 out]
                n381 = property on="Freq/Period" class="Bool (strict)"(error in=w430, "Visible"=w439) -> (error out=w442:errorcluster)  [unwired: 1 in, 1 out]
                n382 = property on="DutyStr" class="Str"("Visible"=TRUE) -> ()  [unwired: 2 in, 2 out]
                n383 = property on="Ampl/HighL" class="Bool (strict)"(error in=w442, "Visible"=w439) -> (error out=w441:errorcluster)  [unwired: 1 in, 1 out]
                n384 = property on="Ampl-HighL" class="Str"(error in=w445, "Visible"=w439) -> (error out=w444:errorcluster)  [unwired: 1 in, 1 out]
                n385 = property on="Offset/LowL" class="Bool (strict)"(error in=w441, "Visible"=w439) -> (error out=w429:errorcluster)  [unwired: 1 in, 1 out]
                n386 = property on="Offset-LowL" class="Str"(error in=w444, "Visible"=w439) -> (error out=w443:errorcluster)  [unwired: 1 in, 1 out]
                n387 = property on="PhaseStr" class="Str"(error in=w443, "Visible"=w439) -> (error out=w435:errorcluster)  [unwired: 1 in, 1 out]
                n388 = property on="Freq" class="DigNum (strict)"(error in=w435, "Visible"=w425) -> (error out=w434:errorcluster)  [unwired: 1 in, 1 out]
                n389 = property on="Offset" class="DigNum (strict)"(error in=w429, "Visible"=w425) -> (error out=w431:errorcluster)  [unwired: 1 in, 1 out]
                n390 = property on="OK" class="Bool (strict)"(error in=w430, "Visible"=w425) -> ()  [unwired: 1 in, 2 out]
                n391 = property on="Sine" class="Bool (strict)"(error in=w430, "Visible"=w425) -> (error out=w438:errorcluster)  [unwired: 1 in, 1 out]
                n392 = property on="Noise" class="Bool (strict)"(error in=w430, "Visible"=w425) -> ()  [unwired: 1 in, 2 out]
                n393 = property on="Period" class="DigNum (strict)"(error in=w434, "Visible"=w425) -> (error out=w433:errorcluster)  [unwired: 1 in, 1 out]
                n394 = property on="LowL" class="DigNum (strict)"(error in=w431, "Visible"=w425) -> (error out=w432:errorcluster)  [unwired: 1 in, 1 out]
                n395 = property on="Square" class="Bool (strict)"(error in=w438, "Visible"=w425) -> (error out=w437:errorcluster)  [unwired: 1 in, 1 out]
                n396 = property on="Ampl" class="DigNum (strict)"(error in=w433, "Visible"=w425) -> (error out=w440:errorcluster)  [unwired: 1 in, 1 out]
                n397 = property on="PhaseDBL" class="DigNum (strict)"(error in=w432, "Visible"=w425) -> ()  [unwired: 1 in, 2 out]
                n398 = property on="Ramp" class="Bool (strict)"(error in=w437, "Visible"=w425) -> (error out=w436:errorcluster)  [unwired: 1 in, 1 out]
                n399 = property on="HighL" class="DigNum (strict)"(error in=w440, "Visible"=w425) -> ()  [unwired: 1 in, 2 out]
                n400 = property on="DutyDBL" class="DigNum (strict)"("Visible"=w425) -> ()  [unwired: 2 in, 2 out]
                n401 = property on="Pulse" class="Bool (strict)"(error in=w436, "Visible"=w425) -> ()  [unwired: 1 in, 2 out]
                n402 = property on="OK" class="Bool (strict)"("Visible"=w425) -> (error out=w423:errorcluster)  [unwired: 2 in, 1 out]
                n403 = property on="OK" class="Bool (strict)"(error in=w423, "Value"=w425) -> (error out=w424:errorcluster)  [unwired: 1 in, 1 out]
              }
              frame False {
                w462 = TRUE ("Visible")
                w448 = FALSE ("Visible")
                n404 = property on="Freq-Period" class="Str"(error in=w453, "Visible"=w462) -> (error out=w468:errorcluster)  [unwired: 1 in, 1 out]
                n405 = property on="Freq/Period" class="Bool (strict)"(error in=w453, "Visible"=w462) -> (error out=w465:errorcluster)  [unwired: 1 in, 1 out]
                n406 = property on="Slider" class="Bool (strict)"("Visible"=TRUE) -> ()  [unwired: 2 in, 2 out]
                n407 = property on="DutyStr" class="Str"("Visible"=FALSE) -> ()  [unwired: 2 in, 2 out]
                n408 = property on="Ampl/HighL" class="Bool (strict)"(error in=w465, "Visible"=w462) -> (error out=w464:errorcluster)  [unwired: 1 in, 1 out]
                n409 = property on="Ampl-HighL" class="Str"(error in=w468, "Visible"=w462) -> (error out=w467:errorcluster)  [unwired: 1 in, 1 out]
                n410 = property on="Offset/LowL" class="Bool (strict)"(error in=w464, "Visible"=w462) -> (error out=w452:errorcluster)  [unwired: 1 in, 1 out]
                n411 = property on="Offset-LowL" class="Str"(error in=w467, "Visible"=w462) -> (error out=w466:errorcluster)  [unwired: 1 in, 1 out]
                n412 = property on="PhaseStr" class="Str"(error in=w466, "Visible"=w462) -> (error out=w458:errorcluster)  [unwired: 1 in, 1 out]
                n413 = property on="Freq" class="DigNum (strict)"(error in=w458, "Visible"=w448) -> (error out=w457:errorcluster)  [unwired: 1 in, 1 out]
                n414 = property on="Offset" class="DigNum (strict)"(error in=w452, "Visible"=w448) -> (error out=w454:errorcluster)  [unwired: 1 in, 1 out]
                n415 = property on="OK" class="Bool (strict)"(error in=w453, "Visible"=w448) -> ()  [unwired: 1 in, 2 out]
                n416 = property on="Sine" class="Bool (strict)"(error in=w453, "Visible"=w448) -> (error out=w461:errorcluster)  [unwired: 1 in, 1 out]
                n417 = property on="Noise" class="Bool (strict)"(error in=w453, "Visible"=w448) -> ()  [unwired: 1 in, 2 out]
                n418 = property on="Period" class="DigNum (strict)"(error in=w457, "Visible"=w448) -> (error out=w456:errorcluster)  [unwired: 1 in, 1 out]
                n419 = property on="LowL" class="DigNum (strict)"(error in=w454, "Visible"=w448) -> (error out=w455:errorcluster)  [unwired: 1 in, 1 out]
                n420 = property on="Square" class="Bool (strict)"(error in=w461, "Visible"=w448) -> (error out=w460:errorcluster)  [unwired: 1 in, 1 out]
                n421 = property on="Ampl" class="DigNum (strict)"(error in=w456, "Visible"=w448) -> (error out=w463:errorcluster)  [unwired: 1 in, 1 out]
                n422 = property on="PhaseDBL" class="DigNum (strict)"(error in=w455, "Visible"=w448) -> ()  [unwired: 1 in, 2 out]
                n423 = property on="Ramp" class="Bool (strict)"(error in=w460, "Visible"=w448) -> (error out=w459:errorcluster)  [unwired: 1 in, 1 out]
                n424 = property on="OK" class="Bool (strict)"("Visible"=w448) -> (error out=w446:errorcluster)  [unwired: 2 in, 1 out]
                n425 = property on="HighL" class="DigNum (strict)"(error in=w463, "Visible"=w448) -> ()  [unwired: 1 in, 2 out]
                n426 = property on="DutyDBL" class="DigNum (strict)"("Visible"=w448) -> ()  [unwired: 2 in, 2 out]
                n427 = property on="Pulse" class="Bool (strict)"(error in=w459, "Visible"=w448) -> ()  [unwired: 1 in, 2 out]
                n428 = property on="OK" class="Bool (strict)"(error in=w446, "Value"=w448) -> (error out=w447:errorcluster)  [unwired: 1 in, 1 out]
              }
            }
          }
          frame 4 {
            n429 = case shown="False" w472 {
              tunnel: w471 -> [w481 w504]
              tunnel: ["Home_Ramp_2.bmp" "Home_Ramp_1.bmp"] -> w470
              tunnel: [w474 w497] -> w469
              frame True {
                w489 = FALSE ("Visible")
                w476 = FALSE ("Visible")
                n430 = property on="Freq-Period" class="Str"(error in=w481, "Visible"=w489) -> (error out=w495:errorcluster)  [unwired: 1 in, 1 out]
                n431 = property on="Freq/Period" class="Bool (strict)"(error in=w481, "Visible"=w489) -> (error out=w492:errorcluster)  [unwired: 1 in, 1 out]
                n432 = property on="DutyStr" class="Str"("Visible"=FALSE) -> ()  [unwired: 2 in, 2 out]
                n433 = property on="Slider" class="Bool (strict)"("Visible"=TRUE) -> ()  [unwired: 2 in, 2 out]
                n434 = property on="Ampl/HighL" class="Bool (strict)"(error in=w492, "Visible"=w489) -> (error out=w491:errorcluster)  [unwired: 1 in, 1 out]
                n435 = property on="Ampl-HighL" class="Str"(error in=w495, "Visible"=w489) -> (error out=w494:errorcluster)  [unwired: 1 in, 1 out]
                n436 = property on="Offset/LowL" class="Bool (strict)"(error in=w491, "Visible"=w489) -> (error out=w480:errorcluster)  [unwired: 1 in, 1 out]
                n437 = property on="Offset-LowL" class="Str"(error in=w494, "Visible"=w489) -> (error out=w493:errorcluster)  [unwired: 1 in, 1 out]
                n438 = property on="PhaseStr" class="Str"(error in=w493, "Visible"=w489) -> (error out=w485:errorcluster)  [unwired: 1 in, 1 out]
                n439 = property on="Freq" class="DigNum (strict)"(error in=w485, "Visible"=w476) -> (error out=w484:errorcluster)  [unwired: 1 in, 1 out]
                n440 = property on="Offset" class="DigNum (strict)"(error in=w480, "Visible"=w476) -> (error out=w482:errorcluster)  [unwired: 1 in, 1 out]
                n441 = property on="OK" class="Bool (strict)"(error in=w481, "Visible"=w476) -> ()  [unwired: 1 in, 2 out]
                n442 = property on="Sine" class="Bool (strict)"(error in=w481, "Visible"=w476) -> (error out=w488:errorcluster)  [unwired: 1 in, 1 out]
                n443 = property on="Noise" class="Bool (strict)"(error in=w481, "Visible"=w476) -> ()  [unwired: 1 in, 2 out]
                n444 = property on="Period" class="DigNum (strict)"(error in=w484, "Visible"=w476) -> (error out=w483:errorcluster)  [unwired: 1 in, 1 out]
                n445 = property on="LowL" class="DigNum (strict)"(error in=w482, "Visible"=w476) -> (error out=w477:errorcluster)  [unwired: 1 in, 1 out]
                n446 = property on="Square" class="Bool (strict)"(error in=w488, "Visible"=w476) -> (error out=w487:errorcluster)  [unwired: 1 in, 1 out]
                n447 = property on="Ampl" class="DigNum (strict)"(error in=w483, "Visible"=w476) -> (error out=w490:errorcluster)  [unwired: 1 in, 1 out]
                n448 = property on="PhaseDBL" class="DigNum (strict)"(error in=w477, "Visible"=w476) -> ()  [unwired: 1 in, 2 out]
                n449 = property on="Ramp" class="Bool (strict)"(error in=w487, "Visible"=w476) -> (error out=w486:errorcluster)  [unwired: 1 in, 1 out]
                n450 = property on="OK" class="Bool (strict)"("Visible"=w476) -> (error out=w473:errorcluster)  [unwired: 2 in, 1 out]
                n451 = property on="HighL" class="DigNum (strict)"(error in=w490, "Visible"=w476) -> ()  [unwired: 1 in, 2 out]
                n452 = property on="DutyDBL" class="DigNum (strict)"(error in=w477, "Visible"=w476) -> ()  [unwired: 1 in, 2 out]
                n453 = property on="Pulse" class="Bool (strict)"(error in=w486, "Visible"=w476) -> ()  [unwired: 1 in, 2 out]
                n454 = property on="OK" class="Bool (strict)"(error in=w473, "Value"=w476) -> (error out=w474:errorcluster)  [unwired: 1 in, 1 out]
              }
              frame False {
                w513 = TRUE ("Visible")
                w499 = FALSE ("Visible")
                n455 = property on="Freq-Period" class="Str"(error in=w504, "Visible"=w513) -> (error out=w519:errorcluster)  [unwired: 1 in, 1 out]
                n456 = property on="Freq/Period" class="Bool (strict)"(error in=w504, "Visible"=w513) -> (error out=w516:errorcluster)  [unwired: 1 in, 1 out]
                n457 = property on="DutyStr" class="Str"("Visible"=FALSE) -> ()  [unwired: 2 in, 2 out]
                n458 = property on="Slider" class="Bool (strict)"("Visible"=TRUE) -> ()  [unwired: 2 in, 2 out]
                n459 = property on="Ampl/HighL" class="Bool (strict)"(error in=w516, "Visible"=w513) -> (error out=w515:errorcluster)  [unwired: 1 in, 1 out]
                n460 = property on="Ampl-HighL" class="Str"(error in=w519, "Visible"=w513) -> (error out=w518:errorcluster)  [unwired: 1 in, 1 out]
                n461 = property on="Offset/LowL" class="Bool (strict)"(error in=w515, "Visible"=w513) -> (error out=w503:errorcluster)  [unwired: 1 in, 1 out]
                n462 = property on="Offset-LowL" class="Str"(error in=w518, "Visible"=w513) -> (error out=w517:errorcluster)  [unwired: 1 in, 1 out]
                n463 = property on="PhaseStr" class="Str"(error in=w517, "Visible"=w513) -> (error out=w509:errorcluster)  [unwired: 1 in, 1 out]
                n464 = property on="Freq" class="DigNum (strict)"(error in=w509, "Visible"=w499) -> (error out=w508:errorcluster)  [unwired: 1 in, 1 out]
                n465 = property on="Offset" class="DigNum (strict)"(error in=w503, "Visible"=w499) -> (error out=w505:errorcluster)  [unwired: 1 in, 1 out]
                n466 = property on="OK" class="Bool (strict)"(error in=w504, "Visible"=w499) -> ()  [unwired: 1 in, 2 out]
                n467 = property on="Sine" class="Bool (strict)"(error in=w504, "Visible"=w499) -> (error out=w512:errorcluster)  [unwired: 1 in, 1 out]
                n468 = property on="Noise" class="Bool (strict)"(error in=w504, "Visible"=w499) -> ()  [unwired: 1 in, 2 out]
                n469 = property on="Period" class="DigNum (strict)"(error in=w508, "Visible"=w499) -> (error out=w507:errorcluster)  [unwired: 1 in, 1 out]
                n470 = property on="LowL" class="DigNum (strict)"(error in=w505, "Visible"=w499) -> (error out=w506:errorcluster)  [unwired: 1 in, 1 out]
                n471 = property on="Square" class="Bool (strict)"(error in=w512, "Visible"=w499) -> (error out=w511:errorcluster)  [unwired: 1 in, 1 out]
                n472 = property on="Ampl" class="DigNum (strict)"(error in=w507, "Visible"=w499) -> (error out=w514:errorcluster)  [unwired: 1 in, 1 out]
                n473 = property on="PhaseDBL" class="DigNum (strict)"(error in=w506, "Visible"=w499) -> (error out=w501:errorcluster)  [unwired: 1 in, 1 out]
                n474 = property on="Ramp" class="Bool (strict)"(error in=w511, "Visible"=w499) -> (error out=w510:errorcluster)  [unwired: 1 in, 1 out]
                n475 = property on="OK" class="Bool (strict)"("Visible"=w499) -> (error out=w496:errorcluster)  [unwired: 2 in, 1 out]
                n476 = property on="HighL" class="DigNum (strict)"(error in=w514, "Visible"=w499) -> ()  [unwired: 1 in, 2 out]
                n477 = property on="DutyDBL" class="DigNum (strict)"(error in=w501, "Visible"=w499) -> ()  [unwired: 1 in, 2 out]
                n478 = property on="Pulse" class="Bool (strict)"(error in=w510, "Visible"=w499) -> ()  [unwired: 1 in, 2 out]
                n479 = property on="OK" class="Bool (strict)"(error in=w496, "Value"=w499) -> (error out=w497:errorcluster)  [unwired: 1 in, 1 out]
              }
            }
          }
          frame 8 {
            n480 = case shown="True" w523 {
              tunnel: w522 -> [w532 w556]
              tunnel: ["Home_Pulse_2.bmp" "Home_Pulse_1.bmp"] -> w521
              tunnel: [w525 w549] -> w520
              frame True {
                w541 = FALSE ("Visible")
                w526 = FALSE ("Visible")
                n481 = property on="Freq-Period" class="Str"(error in=w532, "Visible"=w541) -> (error out=w547:errorcluster)  [unwired: 1 in, 1 out]
                n482 = property on="Freq/Period" class="Bool (strict)"(error in=w532, "Visible"=w541) -> (error out=w544:errorcluster)  [unwired: 1 in, 1 out]
                n483 = property on="DutyStr" class="Str"("Visible"=TRUE) -> ()  [unwired: 2 in, 2 out]
                n484 = property on="Slider" class="Bool (strict)"("Visible"=TRUE) -> ()  [unwired: 2 in, 2 out]
                n485 = property on="Ampl/HighL" class="Bool (strict)"(error in=w544, "Visible"=w541) -> (error out=w543:errorcluster)  [unwired: 1 in, 1 out]
                n486 = property on="Ampl-HighL" class="Str"(error in=w547, "Visible"=w541) -> (error out=w546:errorcluster)  [unwired: 1 in, 1 out]
                n487 = property on="Offset/LowL" class="Bool (strict)"(error in=w543, "Visible"=w541) -> (error out=w531:errorcluster)  [unwired: 1 in, 1 out]
                n488 = property on="Offset-LowL" class="Str"(error in=w546, "Visible"=w541) -> (error out=w545:errorcluster)  [unwired: 1 in, 1 out]
                n489 = property on="PhaseStr" class="Str"(error in=w545, "Visible"=w541) -> (error out=w537:errorcluster)  [unwired: 1 in, 1 out]
                n490 = property on="Freq" class="DigNum (strict)"(error in=w537, "Visible"=w526) -> (error out=w536:errorcluster)  [unwired: 1 in, 1 out]
                n491 = property on="Offset" class="DigNum (strict)"(error in=w531, "Visible"=w526) -> (error out=w533:errorcluster)  [unwired: 1 in, 1 out]
                n492 = property on="OK" class="Bool (strict)"(error in=w532, "Visible"=w526) -> ()  [unwired: 1 in, 2 out]
                n493 = property on="Sine" class="Bool (strict)"(error in=w532, "Visible"=w526) -> (error out=w540:errorcluster)  [unwired: 1 in, 1 out]
                n494 = property on="Noise" class="Bool (strict)"(error in=w532, "Visible"=w526) -> ()  [unwired: 1 in, 2 out]
                n495 = property on="Period" class="DigNum (strict)"(error in=w536, "Visible"=w526) -> (error out=w535:errorcluster)  [unwired: 1 in, 1 out]
                n496 = property on="LowL" class="DigNum (strict)"(error in=w533, "Visible"=w526) -> (error out=w534:errorcluster)  [unwired: 1 in, 1 out]
                n497 = property on="Square" class="Bool (strict)"(error in=w540, "Visible"=w526) -> (error out=w539:errorcluster)  [unwired: 1 in, 1 out]
                n498 = property on="Ampl" class="DigNum (strict)"(error in=w535, "Visible"=w526) -> (error out=w542:errorcluster)  [unwired: 1 in, 1 out]
                n499 = property on="PhaseDBL" class="DigNum (strict)"(error in=w534, "Visible"=w526) -> (error out=w528:errorcluster)  [unwired: 1 in, 1 out]
                n500 = property on="OK" class="Bool (strict)"("Visible"=w526) -> (error out=w524:errorcluster)  [unwired: 2 in, 1 out]
                n501 = property on="Ramp" class="Bool (strict)"(error in=w539, "Visible"=w526) -> (error out=w538:errorcluster)  [unwired: 1 in, 1 out]
                n502 = property on="HighL" class="DigNum (strict)"(error in=w542, "Visible"=w526) -> ()  [unwired: 1 in, 2 out]
                n503 = property on="DutyDBL" class="DigNum (strict)"(error in=w528, "Visible"=w526) -> ()  [unwired: 1 in, 2 out]
                n504 = property on="Pulse" class="Bool (strict)"(error in=w538, "Visible"=w526) -> ()  [unwired: 1 in, 2 out]
                n505 = property on="OK" class="Bool (strict)"(error in=w524, "Value"=w526) -> (error out=w525:errorcluster)  [unwired: 1 in, 1 out]
              }
              frame False {
                w564 = TRUE ("Visible")
                w551 = FALSE ("Visible")
                n506 = property on="Freq-Period" class="Str"(error in=w556, "Visible"=w564) -> (error out=w570:errorcluster)  [unwired: 1 in, 1 out]
                n507 = property on="Freq/Period" class="Bool (strict)"(error in=w556, "Visible"=w564) -> (error out=w567:errorcluster)  [unwired: 1 in, 1 out]
                n508 = property on="DutyStr" class="Str"("Visible"=FALSE) -> ()  [unwired: 2 in, 2 out]
                n509 = property on="Slider" class="Bool (strict)"("Visible"=TRUE) -> ()  [unwired: 2 in, 2 out]
                n510 = property on="Ampl/HighL" class="Bool (strict)"(error in=w567, "Visible"=w564) -> (error out=w566:errorcluster)  [unwired: 1 in, 1 out]
                n511 = property on="Ampl-HighL" class="Str"(error in=w570, "Visible"=w564) -> (error out=w569:errorcluster)  [unwired: 1 in, 1 out]
                n512 = property on="Offset/LowL" class="Bool (strict)"(error in=w566, "Visible"=w564) -> (error out=w555:errorcluster)  [unwired: 1 in, 1 out]
                n513 = property on="Offset-LowL" class="Str"(error in=w569, "Visible"=w564) -> (error out=w568:errorcluster)  [unwired: 1 in, 1 out]
                n514 = property on="PhaseStr" class="Str"(error in=w568, "Visible"=w564) -> (error out=w560:errorcluster)  [unwired: 1 in, 1 out]
                n515 = property on="Freq" class="DigNum (strict)"(error in=w560, "Visible"=w551) -> (error out=w559:errorcluster)  [unwired: 1 in, 1 out]
                n516 = property on="Offset" class="DigNum (strict)"(error in=w555, "Visible"=w551) -> (error out=w557:errorcluster)  [unwired: 1 in, 1 out]
                n517 = property on="OK" class="Bool (strict)"(error in=w556, "Visible"=w551) -> ()  [unwired: 1 in, 2 out]
                n518 = property on="Sine" class="Bool (strict)"(error in=w556, "Visible"=w551) -> (error out=w563:errorcluster)  [unwired: 1 in, 1 out]
                n519 = property on="Noise" class="Bool (strict)"(error in=w556, "Visible"=w551) -> ()  [unwired: 1 in, 2 out]
                n520 = property on="Period" class="DigNum (strict)"(error in=w559, "Visible"=w551) -> (error out=w558:errorcluster)  [unwired: 1 in, 1 out]
                n521 = property on="LowL" class="DigNum (strict)"(error in=w557, "Visible"=w551) -> (error out=w552:errorcluster)  [unwired: 1 in, 1 out]
                n522 = property on="Square" class="Bool (strict)"(error in=w563, "Visible"=w551) -> (error out=w562:errorcluster)  [unwired: 1 in, 1 out]
                n523 = property on="Ampl" class="DigNum (strict)"(error in=w558, "Visible"=w551) -> (error out=w565:errorcluster)  [unwired: 1 in, 1 out]
                n524 = property on="PhaseDBL" class="DigNum (strict)"(error in=w552, "Visible"=w551) -> ()  [unwired: 1 in, 2 out]
                n525 = property on="Ramp" class="Bool (strict)"(error in=w562, "Visible"=w551) -> (error out=w561:errorcluster)  [unwired: 1 in, 1 out]
                n526 = property on="OK" class="Bool (strict)"("Visible"=w551) -> (error out=w548:errorcluster)  [unwired: 2 in, 1 out]
                n527 = property on="HighL" class="DigNum (strict)"(error in=w565, "Visible"=w551) -> ()  [unwired: 1 in, 2 out]
                n528 = property on="DutyDBL" class="DigNum (strict)"(error in=w552, "Visible"=w551) -> ()  [unwired: 1 in, 2 out]
                n529 = property on="Pulse" class="Bool (strict)"(error in=w561, "Visible"=w551) -> ()  [unwired: 1 in, 2 out]
                n530 = property on="OK" class="Bool (strict)"(error in=w548, "Value"=w551) -> (error out=w549:errorcluster)  [unwired: 1 in, 1 out]
              }
            }
          }
          frame 16 {
            w579 = FALSE ("Visible")
            w573 = FALSE ("Visible")
            w574 = TRUE ("Visible")
            n531 = property on="Freq/Period" class="Bool (strict)"(error in=w576, "Visible"=w574) -> (error out=w581:errorcluster)  [unwired: 1 in, 1 out]
            n532 = property on="DutyStr" class="Str"(error in=w576, "Visible"=w573) -> (error out=w571:errorcluster)  [unwired: 1 in, 1 out]
            n533 = property on="Slider" class="Bool (strict)"(error in=w576, "Visible"=FALSE) -> ()  [unwired: 1 in, 2 out]
            n534 = property on="Ampl/HighL" class="Bool (strict)"(error in=w581, "Visible"=w574) -> (error out=w580:errorcluster)  [unwired: 1 in, 1 out]
            n535 = property on="Freq-Period" class="Str"(error in=w571, "Visible"=w573) -> (error out=w572:errorcluster)  [unwired: 1 in, 1 out]
            n536 = property on="Ampl-HighL" class="Str"(error in=w576, "Visible"=w574) -> (error out=w582:errorcluster)  [unwired: 1 in, 1 out]
            n537 = property on="Offset/LowL" class="Bool (strict)"(error in=w580, "Visible"=w574) -> ()  [unwired: 1 in, 2 out]
            n538 = property on="PhaseStr" class="Str"(error in=w572, "Visible"=w573) -> ()  [unwired: 1 in, 2 out]
            n539 = property on="Offset-LowL" class="Str"(error in=w582, "Visible"=w574) -> (error out=w575:errorcluster)  [unwired: 1 in, 1 out]
            n540 = property on="Freq" class="DigNum (strict)"(error in=w575, "Visible"=w579) -> (error out=w586:errorcluster)  [unwired: 1 in, 1 out]
            n541 = property on="DutyDBL" class="DigNum (strict)"("Visible"=w579) -> ()  [unwired: 2 in, 2 out]
            n542 = property on="Period" class="DigNum (strict)"(error in=w586, "Visible"=w579) -> (error out=w583:errorcluster)  [unwired: 1 in, 1 out]
            n543 = property on="Offset" class="DigNum (strict)"(error in=w583, "Visible"=w579) -> (error out=w584:errorcluster)  [unwired: 1 in, 1 out]
            n544 = property on="PhaseDBL" class="DigNum (strict)"(error in=w583, "Visible"=w579) -> ()  [unwired: 1 in, 2 out]
            n545 = property on="Ampl" class="DigNum (strict)"(error in=w583, "Visible"=w579) -> (error out=w585:errorcluster)  [unwired: 1 in, 1 out]
            n546 = property on="LowL" class="DigNum (strict)"(error in=w584, "Visible"=w579) -> ()  [unwired: 1 in, 2 out]
            n547 = property on="HighL" class="DigNum (strict)"(error in=w585, "Visible"=w579) -> ()  [unwired: 1 in, 2 out]
            n548 = property on="OK" class="Bool (strict)"("Visible"=w579) -> (error out=w577:errorcluster)  [unwired: 2 in, 1 out]
            n549 = property on="OK" class="Bool (strict)"(error in=w577, "Value"=w579) -> (error out=w578:errorcluster)  [unwired: 1 in, 1 out]
          }
        }
        n550 = Build Path(base path=w397, name or relative path=w386) -> (appended path=w396:path)
        n551 = call "RDG822 Update Screen.vi"("error in"=w385, "Path to file"=w396) -> ("error out"=w393:errorcluster, "Screen"=w395:picture)  [unwired: 8 in]
        n552 = local write "Screen"(w395) -> ()
        n553 = stacked-sequence {
          tunnel: [_ _ w697 _ _] -> w390
          tunnel: [_ w680 _ _ _] -> w391
          tunnel: [w590 _ _ _ _] -> w392
          tunnel: w400 -> [w591 _ _ _ _]
          tunnel: w399 -> [_ w679 _ _ _]
          tunnel: w398 -> [_ _ w696 _ _]
          tunnel: [_ w678 _ _ _] -> w394
          tunnel: w393 -> [_ w678 _ _ _]
          tunnel: [_ _ _ w721 _] -> w389
          tunnel: [_ _ _ _ w744] -> w388
          tunnel: w382 -> [w589 _ _ _ _]
          frame #0 {
            n554 = case shown="1, Default" w589 {
              tunnel: w591 -> [w592 w614 w630 w647 w663]
              tunnel: [w593 w615 w631 w646 w662] -> w590
              frame 1, Default {
                n555 = case shown="False" w592 {
                  tunnel: [w600 w610] -> w593
                  frame False {
                    n556 = local read "Freq"() -> (w596:dbl)
                    n557 = In Range and Coerce(upper limit=25000.0, x=w596, lower limit=1e-09 ("t")) -> (coerced(x)=w594:dbl, In Range?=w595:bool)
                    n558 = case shown="False" w595 {
                      frame False {
                        n559 = One Button Dialog(message="Frequency can`t be less than 1 uHz\nor more  than 25 MHz!") -> ()  [unwired: 1 in, 1 out]
                      }
                      frame True {
                      }
                    }
                    n560 = local write "Freq"(w594) -> ()
                    n561 = Number To Fractional String(number=w594, precision (6)=i16 9) -> (F-format string=w599:string)  [unwired: 2 in]
                    n562 = Concatenate Strings(w599, " kHz" ("string")) -> (w600:string)
                  }
                  frame True {
                    n563 = local read "Period"() -> (w604:dbl)
                    n564 = In Range and Coerce(upper limit=10000000000.0, x=w604, lower limit=4e-05 ("t")) -> (coerced(x)=w605:dbl, In Range?=w606:bool)
                    n565 = case shown="False" w606 {
                      frame False {
                        n566 = One Button Dialog(message="Period can`t be less than 40 ns or more  than 1 Ms!") -> ()  [unwired: 1 in, 1 out]
                      }
                      frame True {
                      }
                    }
                    n567 = local write "Period"(w605) -> ()
                    n568 = Number To Fractional String(number=w605, precision (6)=i16 7) -> (F-format string=w609:string)  [unwired: 2 in]
                    n569 = Concatenate Strings(w609, " ms" ("string")) -> (w610:string)
                  }
                }
              }
              frame 2 {
                n570 = case shown="False" w614 {
                  tunnel: [w617 w624] -> w615
                  frame False {
                    n571 = local read "Freq"() -> (w620:dbl)
                    n572 = Divide(x=1000.0, y=w620) -> (x/y=w619:dbl)
                    n573 = Number To Fractional String(number=w620, precision (6)=i16 6) -> (F-format string=w616:string)  [unwired: 2 in]
                    n574 = local write "Period"(w619) -> ()
                    n575 = Concatenate Strings(w616, " Hz" ("string")) -> (w617:string)
                  }
                  frame True {
                    n576 = local read "Period"() -> (w627:dbl)
                    n577 = Divide(x=1000.0, y=w627) -> (x/y=w626:dbl)
                    n578 = Number To Fractional String(number=w627, precision (6)=i16 7) -> (F-format string=w623:string)  [unwired: 2 in]
                    n579 = local write "Freq"(w626) -> ()
                    n580 = Concatenate Strings(w623, " ms" ("string")) -> (w624:string)
                  }
                }
              }
              frame 4 {
                n581 = case shown="False" w630 {
                  tunnel: [w633 w640] -> w631
                  frame False {
                    n582 = local read "Freq"() -> (w636:dbl)
                    n583 = Divide(x=1000.0, y=w636) -> (x/y=w635:dbl)
                    n584 = Number To Fractional String(number=w636, precision (6)=i16 6) -> (F-format string=w632:string)  [unwired: 2 in]
                    n585 = local write "Period"(w635) -> ()
                    n586 = Concatenate Strings(w632, " Hz" ("string")) -> (w633:string)
                  }
                  frame True {
                    n587 = local read "Period"() -> (w643:dbl)
                    n588 = Divide(x=1000.0, y=w643) -> (x/y=w642:dbl)
                    n589 = Number To Fractional String(number=w643, precision (6)=i16 7) -> (F-format string=w639:string)  [unwired: 2 in]
                    n590 = local write "Freq"(w642) -> ()
                    n591 = Concatenate Strings(w639, " ms" ("string")) -> (w640:string)
                  }
                }
              }
              frame 8 {
                n592 = case shown="False" w647 {
                  tunnel: [w649 w656] -> w646
                  frame False {
                    n593 = local read "Freq"() -> (w652:dbl)
                    n594 = Divide(x=1000.0, y=w652) -> (x/y=w651:dbl)
                    n595 = Number To Fractional String(number=w652, precision (6)=i16 6) -> (F-format string=w648:string)  [unwired: 2 in]
                    n596 = local write "Period"(w651) -> ()
                    n597 = Concatenate Strings(w648, " Hz" ("string")) -> (w649:string)
                  }
                  frame True {
                    n598 = local read "Period"() -> (w659:dbl)
                    n599 = Divide(x=1000.0, y=w659) -> (x/y=w658:dbl)
                    n600 = Number To Fractional String(number=w659, precision (6)=i16 7) -> (F-format string=w655:string)  [unwired: 2 in]
                    n601 = local write "Freq"(w658) -> ()
                    n602 = Concatenate Strings(w655, " ms" ("string")) -> (w656:string)
                  }
                }
              }
              frame 16 {
                n603 = case shown="True" w663 {
                  tunnel: [w665 w672] -> w662
                  frame False {
                    n604 = local read "Freq"() -> (w668:dbl)
                    n605 = Divide(x=1000.0, y=w668) -> (x/y=w667:dbl)
                    n606 = Number To Fractional String(number=w668, precision (6)=i16 6) -> (F-format string=w664:string)  [unwired: 2 in]
                    n607 = local write "Period"(w667) -> ()
                    n608 = Concatenate Strings(w664, " Hz" ("string")) -> (w665:string)
                  }
                  frame True {
                    n609 = local read "Period"() -> (w675:dbl)
                    n610 = Divide(x=1000.0, y=w675) -> (x/y=w674:dbl)
                    n611 = Number To Fractional String(number=w675, precision (6)=i16 7) -> (F-format string=w671:string)  [unwired: 2 in]
                    n612 = local write "Freq"(w674) -> ()
                    n613 = Concatenate Strings(w671, " ms" ("string")) -> (w672:string)
                  }
                }
              }
            }
          }
          frame #1 {
            n614 = case shown="False" w679 {
              tunnel: [w683 w691] -> w680
              frame False {
                # "Must vary"
                n615 = local read "Ampl"() -> (w688:dbl)
                n616 = In Range and Coerce(upper limit=20.00001, x=w688, lower limit=0.001999 ("t")) -> (coerced(x)=w682:dbl, In Range?=w686:bool)
                n617 = case shown="False" w686 {
                  frame False {
                    n618 = One Button Dialog(message="Amplitude can`t be less than 2 mA\nor more  than 20 A!") -> ()  [unwired: 1 in, 1 out]
                  }
                  frame True {
                  }
                }
                n619 = Number To Fractional String(number=w682, precision (6)=i16 4) -> (F-format string=w684:string)  [unwired: 2 in]
                n620 = local write "Ampl"(w682) -> ()
                n621 = Concatenate Strings(w684, " Vpp" ("string")) -> (w683:string)
              }
              frame True {
                n622 = local read "HighL"() -> (w694:dbl)
                n623 = Number To Fractional String(number=w694, precision (6)=i16 4) -> (F-format string=w692:string)  [unwired: 2 in]
                n624 = Concatenate Strings(w692, " V" ("string")) -> (w691:string)
              }
            }
          }
          frame #2 {
            n625 = case shown="False" w696 {
              tunnel: [w712 w716] -> w697
              frame False {
                n626 = local read "Ampl"() -> (w707:dbl)
                n627 = local read "Ampl"() -> (w702:dbl)
                n628 = Subtract(x=20.00001, y=w707) -> (x-y=w706:dbl)
                n629 = Add(x=-20.00001, y=w702) -> (x+y=w703:dbl)
                n630 = local read "Offset"() -> (w709:dbl)
                n631 = Divide(x=w706, y=2.0) -> (x/y=w704:dbl)
                n632 = Divide(x=w703, y=2.0) -> (x/y=w701:dbl)
                n633 = In Range and Coerce(upper limit=w704, x=w709, lower limit=w701) -> (coerced(x)=w698:dbl, In Range?=w710:bool)
                n634 = case shown="False" w710 {
                  frame False {
                    n635 = One Button Dialog(message="Offset upper and lower limit can`t exceed 20-(Ampl/2) value") -> ()  [unwired: 1 in, 1 out]
                  }
                  frame True {
                  }
                }
                n636 = local write "Offset"(w698) -> ()
                n637 = Number To Fractional String(number=w698, precision (6)=i16 4) -> (F-format string=w711:string)  [unwired: 2 in]
                n638 = Concatenate Strings(w711, " Vdc" ("string")) -> (w712:string)
              }
              frame True {
                n639 = local read "LowL"() -> (w719:dbl)
                n640 = Number To Fractional String(number=w719, precision (6)=i16 4) -> (F-format string=w717:string)  [unwired: 2 in]
                n641 = Concatenate Strings(w717, " V" ("string")) -> (w716:string)
              }
            }
          }
          frame #3 {
            n642 = local read "PhaseDBL"() -> (w725:dbl)
            n643 = while {
              shift-right: [w727] -> w724
              shift-left: w725 -> [w729]
              stop <- w728 stop-if-true
              w730 = 360.0001 ("upper limit")
              n644 = In Range and Coerce(upper limit=w730, x=w729, lower limit=0.0) -> (In Range?=w728:bool)  [unwired: 1 out]
              n645 = case shown="True" w728 {
                tunnel: w730 -> [w735 _]
                tunnel: w729 -> [w733 w742]
                tunnel: [w732 w742] -> w727
                frame False {
                  n646 = Greater?(x=w733, y=w735) -> (0:w734:bool)
                  n647 = case shown="True" w734 {
                    tunnel: w733 -> [w737 w739]
                    tunnel: [w736 w740] -> w732
                    frame False {
                      n648 = Add(x=w737, y=360.0) -> (x+y=w736:dbl)
                    }
                    frame True {
                      n649 = Subtract(x=w739, y=360.0) -> (x-y=w740:dbl)
                    }
                  }
                }
                frame True {
                }
              }
            }
            n650 = Number To Fractional String(number=w724, precision (6)=i16 3) -> (F-format string=w722:string)  [unwired: 2 in]
            n651 = Concatenate Strings(w722, " °" ("string")) -> (w721:string)
          }
          frame #4 {
            n652 = local read "DutyDBL"() -> (w747:dbl)
            n653 = while {
              shift-right: [w749] -> w746
              shift-left: w747 -> [w751]
              stop <- w750 stop-if-true
              w752 = 100.0001 ("upper limit")
              n654 = In Range and Coerce(upper limit=w752, x=w751, lower limit=0.0) -> (In Range?=w750:bool)  [unwired: 1 out]
              n655 = case shown="True" w750 {
                tunnel: w752 -> [w757 _]
                tunnel: w751 -> [w755 w764]
                tunnel: [w754 w764] -> w749
                frame False {
                  n656 = Greater?(x=w755, y=w757) -> (0:w756:bool)
                  n657 = case shown="False" w756 {
                    tunnel: w755 -> [w759 w761]
                    tunnel: [w758 w762] -> w754
                    frame False {
                      n658 = Add(x=w759, y=100.0) -> (x+y=w758:dbl)
                    }
                    frame True {
                      n659 = Subtract(x=w761, y=100.0) -> (x-y=w762:dbl)
                    }
                  }
                }
                frame True {
                }
              }
            }
            n660 = Number To Fractional String(number=w746, precision (6)=i16 3) -> (F-format string=w743:string)  [unwired: 2 in]
            n661 = Concatenate Strings(w743, " %" ("string")) -> (w744:string)
          }
        }
        n662 = local write "error out"(w394) -> ()
        n663 = local write "Freq-Period"(w392) -> ()
        n664 = local write "Ampl-HighL"(w391) -> ()
        n665 = local write "Offset-LowL"(w390) -> ()
        n666 = local write "PhaseStr"(w389) -> ()
        n667 = local write "DutyStr"(w388) -> ()
      }
      event "Freq-Period": Mouse Down {
        w765 = FALSE ("Visible")
        n668 = event-data() -> ()  [unwired: 1 in, 8 out]
        n669 = property on="Freq-Period" class="Str"("Visible"=w765) -> (error out=w782:errorcluster)  [unwired: 2 in, 1 out]
        n670 = property on="Freq/Period" class="Bool (strict)"("Visible"=w765) -> (error out=w781:errorcluster)  [unwired: 2 in, 1 out]
        n671 = property on="Freq" class="DigNum (strict)"("Visible"=w765) -> (error out=w784:errorcluster)  [unwired: 2 in, 1 out]
        n672 = property on="Offset" class="DigNum (strict)"("Visible"=w765) -> (error out=w776:errorcluster)  [unwired: 2 in, 1 out]
        n673 = property on="Ampl-HighL" class="Str"(error in=w782, "Visible"=w765) -> (error out=w778:errorcluster)  [unwired: 1 in, 1 out]
        n674 = property on="Ampl/HighL" class="Bool (strict)"(error in=w781, "Visible"=w765) -> (error out=w777:errorcluster)  [unwired: 1 in, 1 out]
        n675 = property on="Period" class="DigNum (strict)"(error in=w784, "Visible"=w765) -> (error out=w780:errorcluster)  [unwired: 1 in, 1 out]
        n676 = property on="LowL" class="DigNum (strict)"(error in=w776, "Visible"=w765) -> (error out=w773:errorcluster)  [unwired: 1 in, 1 out]
        n677 = property on="Offset-LowL" class="Str"(error in=w778, "Visible"=w765) -> (error out=w775:errorcluster)  [unwired: 1 in, 1 out]
        n678 = property on="Offset/LowL" class="Bool (strict)"(error in=w777, "Visible"=w765) -> (error out=w768:errorcluster)  [unwired: 1 in, 1 out]
        n679 = property on="Ampl" class="DigNum (strict)"(error in=w780, "Visible"=w765) -> (error out=w779:errorcluster)  [unwired: 1 in, 1 out]
        n680 = property on="PhaseDBL" class="DigNum (strict)"(error in=w773, "Visible"=w765) -> (error out=w767:errorcluster)  [unwired: 1 in, 1 out]
        n681 = property on="Slider" class="Bool (strict)"(error in=w768, "Visible"=w765) -> ()  [unwired: 1 in, 2 out]
        n682 = property on="PhaseStr" class="Str"(error in=w775, "Visible"=w765) -> ()  [unwired: 1 in, 2 out]
        n683 = property on="HighL" class="DigNum (strict)"(error in=w779, "Visible"=w765) -> ()  [unwired: 1 in, 2 out]
        n684 = property on="DutyDBL" class="DigNum (strict)"(error in=w767, "Visible"=w765) -> (error out=w766:errorcluster)  [unwired: 1 in, 1 out]
        n685 = case shown="False" w783 {
          tunnel: [w791 w797] -> w772
          tunnel: w785 -> [w789 w795]
          tunnel: w766 -> [w787 w793]
          tunnel: [w786 w792] -> w771
          frame False {
            n686 = property on="Freq" class="DigNum (strict)"(error in=w787, "Visible"=TRUE) -> (error out=w786:errorcluster)  [unwired: 1 in, 1 out]
            n687 = Build Path(base path=w789, name or relative path="Freq.bmp") -> (appended path=w791:path)
          }
          frame True {
            n688 = property on="Period" class="DigNum (strict)"(error in=w793, "Visible"=TRUE) -> (error out=w792:errorcluster)  [unwired: 1 in, 1 out]
            n689 = Build Path(base path=w795, name or relative path="Period.bmp") -> (appended path=w797:path)
          }
        }
        n690 = call "RDG822 Update Screen.vi"("error in"=w771, "Path to file"=w772) -> ("error out"=w770:errorcluster, "Screen"=w769:picture)  [unwired: 8 in]
        n691 = local write "Screen"(w769) -> ()
        n692 = property on="OK" class="Bool (strict)"("Visible"=TRUE) -> ()  [unwired: 2 in, 2 out]
      }
      event "Ampl-HighL": Mouse Down {
        w799 = FALSE ("Visible")
        n693 = event-data() -> ()  [unwired: 1 in, 8 out]
        n694 = property on="Freq-Period" class="Str"("Visible"=w799) -> (error out=w816:errorcluster)  [unwired: 2 in, 1 out]
        n695 = property on="Freq/Period" class="Bool (strict)"("Visible"=w799) -> (error out=w815:errorcluster)  [unwired: 2 in, 1 out]
        n696 = property on="Offset" class="DigNum (strict)"("Visible"=w799) -> (error out=w809:errorcluster)  [unwired: 2 in, 1 out]
        n697 = property on="Freq" class="DigNum (strict)"("Visible"=w799) -> (error out=w817:errorcluster)  [unwired: 2 in, 1 out]
        n698 = property on="Ampl-HighL" class="Str"(error in=w816, "Visible"=w799) -> (error out=w811:errorcluster)  [unwired: 1 in, 1 out]
        n699 = property on="Ampl/HighL" class="Bool (strict)"(error in=w815, "Visible"=w799) -> (error out=w810:errorcluster)  [unwired: 1 in, 1 out]
        n700 = property on="Period" class="DigNum (strict)"(error in=w817, "Visible"=w799) -> (error out=w814:errorcluster)  [unwired: 1 in, 1 out]
        n701 = property on="LowL" class="DigNum (strict)"(error in=w809, "Visible"=w799) -> (error out=w806:errorcluster)  [unwired: 1 in, 1 out]
        n702 = property on="Offset-LowL" class="Str"(error in=w811, "Visible"=w799) -> (error out=w808:errorcluster)  [unwired: 1 in, 1 out]
        n703 = property on="Offset/LowL" class="Bool (strict)"(error in=w810, "Visible"=w799) -> (error out=w801:errorcluster)  [unwired: 1 in, 1 out]
        n704 = property on="Ampl" class="DigNum (strict)"(error in=w814, "Visible"=w799) -> (error out=w812:errorcluster)  [unwired: 1 in, 1 out]
        n705 = property on="PhaseDBL" class="DigNum (strict)"(error in=w806, "Visible"=w799) -> (error out=w800:errorcluster)  [unwired: 1 in, 1 out]
        n706 = property on="PhaseStr" class="Str"(error in=w808, "Visible"=w799) -> ()  [unwired: 1 in, 2 out]
        n707 = property on="Slider" class="Bool (strict)"(error in=w801, "Visible"=w799) -> ()  [unwired: 1 in, 2 out]
        n708 = property on="HighL" class="DigNum (strict)"(error in=w812, "Visible"=w799) -> ()  [unwired: 1 in, 2 out]
        n709 = property on="DutyDBL" class="DigNum (strict)"(error in=w800, "Visible"=w799) -> (error out=w798:errorcluster)  [unwired: 1 in, 1 out]
        n710 = case shown="False" w813 {
          tunnel: [w824 w830] -> w805
          tunnel: w818 -> [w822 w828]
          tunnel: w798 -> [w820 w827]
          tunnel: [w819 w825] -> w804
          frame False {
            n711 = property on="Ampl" class="DigNum (strict)"(error in=w820, "Visible"=TRUE) -> (error out=w819:errorcluster)  [unwired: 1 in, 1 out]
            n712 = Build Path(base path=w822, name or relative path="Ampl.bmp") -> (appended path=w824:path)
          }
          frame True {
            n713 = property on="HighL" class="DigNum (strict)"(error in=w827, "Visible"=TRUE) -> (error out=w825:errorcluster)  [unwired: 1 in, 1 out]
            n714 = Build Path(base path=w828, name or relative path="HighL.bmp") -> (appended path=w830:path)
          }
        }
        n715 = call "RDG822 Update Screen.vi"("error in"=w804, "Path to file"=w805) -> ("error out"=w803:errorcluster, "Screen"=w802:picture)  [unwired: 8 in]
        n716 = local write "Screen"(w802) -> ()
        n717 = property on="OK" class="Bool (strict)"("Visible"=TRUE) -> ()  [unwired: 2 in, 2 out]
      }
      event "Offset-LowL": Mouse Down {
        w831 = FALSE ("Visible")
        n718 = event-data() -> ()  [unwired: 1 in, 8 out]
        n719 = property on="Freq-Period" class="Str"("Visible"=w831) -> (error out=w849:errorcluster)  [unwired: 2 in, 1 out]
        n720 = property on="Freq/Period" class="Bool (strict)"("Visible"=w831) -> (error out=w848:errorcluster)  [unwired: 2 in, 1 out]
        n721 = property on="Freq" class="DigNum (strict)"("Visible"=w831) -> (error out=w850:errorcluster)  [unwired: 2 in, 1 out]
        n722 = property on="Offset" class="DigNum (strict)"("Visible"=w831) -> (error out=w843:errorcluster)  [unwired: 2 in, 1 out]
        n723 = property on="Ampl-HighL" class="Str"(error in=w849, "Visible"=w831) -> (error out=w845:errorcluster)  [unwired: 1 in, 1 out]
        n724 = property on="Ampl/HighL" class="Bool (strict)"(error in=w848, "Visible"=w831) -> (error out=w844:errorcluster)  [unwired: 1 in, 1 out]
        n725 = property on="Period" class="DigNum (strict)"(error in=w850, "Visible"=w831) -> (error out=w847:errorcluster)  [unwired: 1 in, 1 out]
        n726 = property on="LowL" class="DigNum (strict)"(error in=w843, "Visible"=w831) -> (error out=w839:errorcluster)  [unwired: 1 in, 1 out]
        n727 = property on="Offset-LowL" class="Str"(error in=w845, "Visible"=w831) -> (error out=w842:errorcluster)  [unwired: 1 in, 1 out]
        n728 = property on="Offset/LowL" class="Bool (strict)"(error in=w844, "Visible"=w831) -> (error out=w834:errorcluster)  [unwired: 1 in, 1 out]
        n729 = property on="Ampl" class="DigNum (strict)"(error in=w847, "Visible"=w831) -> (error out=w846:errorcluster)  [unwired: 1 in, 1 out]
        n730 = property on="PhaseDBL" class="DigNum (strict)"(error in=w839, "Visible"=w831) -> (error out=w833:errorcluster)  [unwired: 1 in, 1 out]
        n731 = property on="PhaseStr" class="Str"(error in=w842, "Visible"=w831) -> ()  [unwired: 1 in, 2 out]
        n732 = property on="Slider" class="Bool (strict)"(error in=w834, "Visible"=w831) -> ()  [unwired: 1 in, 2 out]
        n733 = property on="HighL" class="DigNum (strict)"(error in=w846, "Visible"=w831) -> ()  [unwired: 1 in, 2 out]
        n734 = property on="DutyDBL" class="DigNum (strict)"(error in=w833, "Visible"=w831) -> (error out=w832:errorcluster)  [unwired: 1 in, 1 out]
        n735 = case shown="False" w841 {
          tunnel: [w857 w863] -> w838
          tunnel: w851 -> [w855 w861]
          tunnel: w832 -> [w853 w860]
          tunnel: [w852 w858] -> w837
          frame False {
            n736 = property on="Offset" class="DigNum (strict)"(error in=w853, "Visible"=TRUE) -> (error out=w852:errorcluster)  [unwired: 1 in, 1 out]
            n737 = Build Path(base path=w855, name or relative path="Offset.bmp") -> (appended path=w857:path)
          }
          frame True {
            n738 = property on="LowL" class="DigNum (strict)"(error in=w860, "Visible"=TRUE) -> (error out=w858:errorcluster)  [unwired: 1 in, 1 out]
            n739 = Build Path(base path=w861, name or relative path="LowL.bmp") -> (appended path=w863:path)
          }
        }
        n740 = call "RDG822 Update Screen.vi"("error in"=w837, "Path to file"=w838) -> ("error out"=w836:errorcluster, "Screen"=w835:picture)  [unwired: 8 in]
        n741 = local write "Screen"(w835) -> ()
        n742 = property on="OK" class="Bool (strict)"("Visible"=TRUE) -> ()  [unwired: 2 in, 2 out]
      }
      event "PhaseStr": Mouse Down {
        w865 = FALSE ("Visible")
        n743 = event-data() -> ()  [unwired: 1 in, 8 out]
        n744 = property on="Freq-Period" class="Str"("Visible"=w865) -> (error out=w883:errorcluster)  [unwired: 2 in, 1 out]
        n745 = property on="Freq/Period" class="Bool (strict)"("Visible"=w865) -> (error out=w882:errorcluster)  [unwired: 2 in, 1 out]
        n746 = property on="Freq" class="DigNum (strict)"("Visible"=w865) -> (error out=w884:errorcluster)  [unwired: 2 in, 1 out]
        n747 = property on="Offset" class="DigNum (strict)"("Visible"=w865) -> (error out=w877:errorcluster)  [unwired: 2 in, 1 out]
        n748 = property on="Ampl-HighL" class="Str"(error in=w883, "Visible"=w865) -> (error out=w879:errorcluster)  [unwired: 1 in, 1 out]
        n749 = property on="Ampl/HighL" class="Bool (strict)"(error in=w882, "Visible"=w865) -> (error out=w878:errorcluster)  [unwired: 1 in, 1 out]
        n750 = property on="Period" class="DigNum (strict)"(error in=w884, "Visible"=w865) -> (error out=w881:errorcluster)  [unwired: 1 in, 1 out]
        n751 = property on="LowL" class="DigNum (strict)"(error in=w877, "Visible"=w865) -> (error out=w872:errorcluster)  [unwired: 1 in, 1 out]
        n752 = property on="Offset-LowL" class="Str"(error in=w879, "Visible"=w865) -> (error out=w876:errorcluster)  [unwired: 1 in, 1 out]
        n753 = property on="Offset/LowL" class="Bool (strict)"(error in=w878, "Visible"=w865) -> (error out=w866:errorcluster)  [unwired: 1 in, 1 out]
        n754 = property on="Ampl" class="DigNum (strict)"(error in=w881, "Visible"=w865) -> (error out=w880:errorcluster)  [unwired: 1 in, 1 out]
        n755 = property on="PhaseDBL" class="DigNum (strict)"(error in=w872, "Visible"=w865) -> ()  [unwired: 1 in, 2 out]
        n756 = property on="PhaseStr" class="Str"(error in=w876, "Visible"=w865) -> ()  [unwired: 1 in, 2 out]
        n757 = property on="Slider" class="Bool (strict)"(error in=w866, "Visible"=w865) -> ()  [unwired: 1 in, 2 out]
        n758 = property on="HighL" class="DigNum (strict)"(error in=w880, "Visible"=w865) -> ()  [unwired: 1 in, 2 out]
        n759 = property on="DutyDBL" class="DigNum (strict)"("Visible"=w865) -> (error out=w864:errorcluster)  [unwired: 2 in, 1 out]
        n760 = property on="PhaseDBL" class="DigNum (strict)"(error in=w864, "Visible"=TRUE) -> (error out=w869:errorcluster)  [unwired: 1 in, 1 out]
        n761 = Build Path(base path=w874, name or relative path="Phase.bmp") -> (appended path=w870:path)
        n762 = call "RDG822 Update Screen.vi"("error in"=w869, "Path to file"=w870) -> ("error out"=w868:errorcluster, "Screen"=w867:picture)  [unwired: 8 in]
        n763 = local write "Screen"(w867) -> ()
        n764 = property on="OK" class="Bool (strict)"("Visible"=TRUE) -> ()  [unwired: 2 in, 2 out]
      }
      event "DutyStr": Mouse Down {
        w886 = FALSE ("Visible")
        n765 = event-data() -> ()  [unwired: 1 in, 8 out]
        n766 = property on="Freq-Period" class="Str"("Visible"=w886) -> (error out=w904:errorcluster)  [unwired: 2 in, 1 out]
        n767 = property on="Freq/Period" class="Bool (strict)"("Visible"=w886) -> (error out=w903:errorcluster)  [unwired: 2 in, 1 out]
        n768 = property on="Freq" class="DigNum (strict)"("Visible"=w886) -> (error out=w905:errorcluster)  [unwired: 2 in, 1 out]
        n769 = property on="Offset" class="DigNum (strict)"("Visible"=w886) -> (error out=w898:errorcluster)  [unwired: 2 in, 1 out]
        n770 = property on="Ampl-HighL" class="Str"(error in=w904, "Visible"=w886) -> (error out=w900:errorcluster)  [unwired: 1 in, 1 out]
        n771 = property on="Ampl/HighL" class="Bool (strict)"(error in=w903, "Visible"=w886) -> (error out=w899:errorcluster)  [unwired: 1 in, 1 out]
        n772 = property on="Period" class="DigNum (strict)"(error in=w905, "Visible"=w886) -> (error out=w902:errorcluster)  [unwired: 1 in, 1 out]
        n773 = property on="LowL" class="DigNum (strict)"(error in=w898, "Visible"=w886) -> (error out=w893:errorcluster)  [unwired: 1 in, 1 out]
        n774 = property on="Offset-LowL" class="Str"(error in=w900, "Visible"=w886) -> (error out=w897:errorcluster)  [unwired: 1 in, 1 out]
        n775 = property on="Offset/LowL" class="Bool (strict)"(error in=w899, "Visible"=w886) -> (error out=w887:errorcluster)  [unwired: 1 in, 1 out]
        n776 = property on="Ampl" class="DigNum (strict)"(error in=w902, "Visible"=w886) -> (error out=w901:errorcluster)  [unwired: 1 in, 1 out]
        n777 = property on="PhaseDBL" class="DigNum (strict)"(error in=w893, "Visible"=w886) -> ()  [unwired: 1 in, 2 out]
        n778 = property on="PhaseStr" class="Str"(error in=w897, "Visible"=w886) -> ()  [unwired: 1 in, 2 out]
        n779 = property on="Slider" class="Bool (strict)"(error in=w887, "Visible"=w886) -> ()  [unwired: 1 in, 2 out]
        n780 = property on="HighL" class="DigNum (strict)"(error in=w901, "Visible"=w886) -> ()  [unwired: 1 in, 2 out]
        n781 = property on="DutyDBL" class="DigNum (strict)"("Visible"=w886) -> (error out=w885:errorcluster)  [unwired: 2 in, 1 out]
        n782 = property on="DutyDBL" class="DigNum (strict)"(error in=w885, "Visible"=TRUE) -> (error out=w890:errorcluster)  [unwired: 1 in, 1 out]
        n783 = Build Path(base path=w895, name or relative path="Duty.bmp") -> (appended path=w891:path)
        n784 = property on="DutyStr" class="Str"("Visible"=w886) -> ()  [unwired: 2 in, 2 out]
        n785 = call "RDG822 Update Screen.vi"("error in"=w890, "Path to file"=w891) -> ("error out"=w889:errorcluster, "Screen"=w888:picture)  [unwired: 8 in]
        n786 = local write "Screen"(w888) -> ()
        n787 = property on="OK" class="Bool (strict)"("Visible"=TRUE) -> ()  [unwired: 2 in, 2 out]
      }
      event "Freq/Period": Value Change {
        n788 = event-data() -> ("NewVal"=w906:bool)  [unwired: 1 in, 5 out]
        n789 = case shown="False" w906 {
          tunnel: [w910 w916] -> w907
          frame False {
            # "Must vary"
            n790 = local read "Period"() -> (w913:dbl)
            n791 = Divide(x=1.0, y=w913) -> (x/y=w911:dbl)
            n792 = Number To Fractional String(number=w911, precision (6)=i16 9) -> (F-format string=w908:string)  [unwired: 2 in]
            n793 = local write "Freq"(w911) -> ()
            n794 = Concatenate Strings(w908, " kHz" ("string")) -> (w910:string)
          }
          frame True {
            # "Must vary"
            n795 = local read "Freq"() -> (w919:dbl)
            n796 = Divide(x=1.0, y=w919) -> (x/y=w918:dbl)
            n797 = local write "Period"(w918) -> ()
            n798 = Number To Fractional String(number=w918, precision (6)=i16 7) -> (F-format string=w915:string)  [unwired: 2 in]
            n799 = Concatenate Strings(w915, " ms" ("string")) -> (w916:string)
          }
        }
        n800 = local write "Freq-Period"(w907) -> ()
      }
      event "Ampl/HighL": Value Change {
        n801 = event-data() -> ("NewVal"=w923:bool)  [unwired: 1 in, 5 out]
        n802 = case shown="True" w923 {
          tunnel: [w933 w941] -> w924
          frame False {
            n803 = local read "HighL"() -> (w928:dbl)
            n804 = local read "LowL"() -> (w927:dbl)
            n805 = Add(x=w928, y=w927) -> (x+y=w930:dbl)
            n806 = Divide(x=w930, y=2.0) -> (x/y=w926:dbl)
            n807 = Number To Fractional String(number=w926, precision (6)=i16 4) -> (F-format string=w931:string)  [unwired: 2 in]
            n808 = local write "Offset"(w926) -> ()
            n809 = Concatenate Strings(w931, " Vdc" ("string")) -> (w933:string)
          }
          frame True {
            n810 = local read "Offset"() -> (w937:dbl)
            n811 = local read "Ampl"() -> (w936:dbl)
            n812 = Divide(x=w936, y=2.0) -> (x/y=w939:dbl)
            n813 = Subtract(x=w937, y=w939) -> (x-y=w938:dbl)
            n814 = local write "LowL"(w938) -> ()
            n815 = Number To Fractional String(number=w938, precision (6)=i16 4) -> (F-format string=w940:string)  [unwired: 2 in]
            n816 = Concatenate Strings(w940, " V" ("string")) -> (w941:string)
          }
        }
        n817 = case shown="False" w923 {
          tunnel: [w948 w957] -> w925
          frame False {
            n818 = local read "HighL"() -> (w946:dbl)
            n819 = local read "LowL"() -> (w945:dbl)
            n820 = Subtract(x=w946, y=w945) -> (x-y=w944:dbl)
            n821 = Number To Fractional String(number=w944, precision (6)=i16 4) -> (F-format string=w947:string)  [unwired: 2 in]
            n822 = local write "Ampl"(w944) -> ()
            n823 = Concatenate Strings(w947, " Vpp" ("string")) -> (w948:string)
          }
          frame True {
            n824 = local read "Offset"() -> (w953:dbl)
            n825 = local read "Ampl"() -> (w954:dbl)
            n826 = Divide(x=w954, y=2.0) -> (x/y=w952:dbl)
            n827 = Add(x=w953, y=w952) -> (x+y=w951:dbl)
            n828 = Number To Fractional String(number=w951, precision (6)=i16 4) -> (F-format string=w956:string)  [unwired: 2 in]
            n829 = local write "HighL"(w951) -> ()
            n830 = Concatenate Strings(w956, " V" ("string")) -> (w957:string)
          }
        }
        n831 = local read "Ampl/HighL"() -> (w922:bool)
        n832 = local write "Offset-LowL"(w924) -> ()
        n833 = local write "Ampl-HighL"(w925) -> ()
        n834 = local write "Offset/LowL"(w922) -> ()
      }
      event "Offset/LowL": Value Change {
        n835 = event-data() -> ("NewVal"=w961:bool)  [unwired: 1 in, 5 out]
        n836 = case shown="False" w961 {
          tunnel: [w971 w979] -> w962
          frame False {
            n837 = local read "HighL"() -> (w966:dbl)
            n838 = local read "LowL"() -> (w965:dbl)
            n839 = Add(x=w966, y=w965) -> (x+y=w968:dbl)
            n840 = Divide(x=w968, y=2.0) -> (x/y=w964:dbl)
            n841 = Number To Fractional String(number=w964, precision (6)=i16 4) -> (F-format string=w969:string)  [unwired: 2 in]
            n842 = local write "Offset"(w964) -> ()
            n843 = Concatenate Strings(w969, " Vdc" ("string")) -> (w971:string)
          }
          frame True {
            n844 = local read "Offset"() -> (w975:dbl)
            n845 = local read "Ampl"() -> (w974:dbl)
            n846 = Divide(x=w974, y=2.0) -> (x/y=w977:dbl)
            n847 = Subtract(x=w975, y=w977) -> (x-y=w976:dbl)
            n848 = local write "LowL"(w976) -> ()
            n849 = Number To Fractional String(number=w976, precision (6)=i16 4) -> (F-format string=w978:string)  [unwired: 2 in]
            n850 = Concatenate Strings(w978, " V" ("string")) -> (w979:string)
          }
        }
        n851 = case shown="False" w961 {
          tunnel: [w986 w995] -> w963
          frame False {
            n852 = local read "HighL"() -> (w984:dbl)
            n853 = local read "LowL"() -> (w983:dbl)
            n854 = Subtract(x=w984, y=w983) -> (x-y=w982:dbl)
            n855 = Number To Fractional String(number=w982, precision (6)=i16 4) -> (F-format string=w985:string)  [unwired: 2 in]
            n856 = local write "Ampl"(w982) -> ()
            n857 = Concatenate Strings(w985, " Vpp" ("string")) -> (w986:string)
          }
          frame True {
            n858 = local read "Offset"() -> (w991:dbl)
            n859 = local read "Ampl"() -> (w992:dbl)
            n860 = Divide(x=w992, y=2.0) -> (x/y=w990:dbl)
            n861 = Add(x=w991, y=w990) -> (x+y=w989:dbl)
            n862 = Number To Fractional String(number=w989, precision (6)=i16 4) -> (F-format string=w994:string)  [unwired: 2 in]
            n863 = local write "HighL"(w989) -> ()
            n864 = Concatenate Strings(w994, " V" ("string")) -> (w995:string)
          }
        }
        n865 = local write "Offset-LowL"(w962) -> ()
        n866 = local write "Ampl-HighL"(w963) -> ()
        n867 = local read "Offset/LowL"() -> (w960:bool)
        n868 = local write "Ampl/HighL"(w960) -> ()
      }
      event "Out1": Mouse Down {
        w1007 = 0 items=["Vpp", "Vrms", "dBm"] ("Amplitude Unit (0: Vpp)")
        w1021 = u16 2 items=["Send", "Read", "Download", "Remove"] ("Send/Read/Download/Remove")
        w1022 = u16 0 items=["Send", "Read", "Download", "Remove"] ("Send/Read/Download/Remove")
        w1010 = FALSE ("Visible")
        w1025 = 1 items=["Channel 1"=1, "Channel 2"=2] ("Output Channel (1: Channel 1)")
        n869 = event-data() -> ()  [unwired: 1 in, 8 out]
        n870 = local read "MenuCont"() -> (w998:u32)
        n871 = case shown="1, Default" w998 {
          tunnel: ["Sine" "Square" "Ramp" "Pulse" "Noise"] -> w999
          frame 1, Default {
          }
          frame 2 {
          }
          frame 4 {
          }
          frame 8 {
          }
          frame 16 {
          }
        }
        n872 = case shown="False" w1044 {
          tunnel: w1043 -> [w1105 _]
          tunnel: w1042 -> [_ w1107]
          tunnel: [w1103 w1106] -> w1005
          frame False {
            # "Freq"
            n873 = Multiply(x=1000.0, y=w1105) -> (x*y=w1103:dbl)
          }
          frame True {
            # "Period"
            n874 = Divide(x=1000.0, y=w1107) -> (x/y=w1106:dbl)
          }
        }
        n875 = case shown="True" w1045 {
          tunnel: w1041 -> [w1094 _]
          tunnel: w1038 -> [_ w1101]
          tunnel: [w1094 w1095] -> w1002
          tunnel: w1039 -> [_ w1100]
          frame False {
          }
          frame True {
            # "High-Low"
            n876 = Subtract(x=w1101, y=w1100) -> (x-y=w1097:dbl)
            n877 = In Range and Coerce(upper limit=20.0000001, x=w1097, lower limit=0.00199999 ("t")) -> (coerced(x)=w1095:dbl, In Range?=w1096:bool)
            n878 = case shown="False" w1096 {
              frame False {
                n879 = One Button Dialog(message="Amplitude can`t be less than 2 mA\nor greater than 20 A!") -> ()  [unwired: 1 in, 1 out]
              }
              frame True {
              }
            }
          }
        }
        n880 = case shown="True" w1040 {
          tunnel: w1004 -> [w1088 _]
          tunnel: w1039 -> [_ w1093]
          tunnel: [w1088 w1089] -> w1003
          tunnel: w1038 -> [_ w1090]
          frame False {
            # "Offset"
          }
          frame True {
            # "HOffset"
            n881 = Add(x=w1090, y=w1093) -> (x+y=w1092:dbl)
            n882 = Divide(x=w1092, y=2.0) -> (x/y=w1089:dbl)
          }
        }
        n883 = while {
          shift-right: [w1072] -> w1006
          shift-left: w1032 -> [w1074]
          stop <- w1073 stop-if-true
          w1075 = 360.0001 ("upper limit")
          # "Phase"
          n884 = In Range and Coerce(upper limit=w1075, x=w1074, lower limit=0.0) -> (In Range?=w1073:bool)  [unwired: 1 out]
          n885 = case shown="False" w1073 {
            tunnel: w1075 -> [w1080 _]
            tunnel: w1074 -> [w1078 w1087]
            tunnel: [w1077 w1087] -> w1072
            frame False {
              n886 = Greater?(x=w1078, y=w1080) -> (0:w1079:bool)
              n887 = case shown="True" w1079 {
                tunnel: w1078 -> [w1082 w1084]
                tunnel: [w1081 w1085] -> w1077
                frame False {
                  n888 = Add(x=w1082, y=360.0) -> (x+y=w1081:dbl)
                }
                frame True {
                  n889 = Subtract(x=w1084, y=360.0) -> (x-y=w1085:dbl)
                }
              }
            }
            frame True {
            }
          }
        }
        n890 = while {
          shift-right: [w1051] -> w1000
          shift-left: w1001 -> [w1053]
          stop <- w1052 stop-if-true
          w1054 = 100.0001 ("upper limit")
          # "Duty"
          n891 = In Range and Coerce(upper limit=w1054, x=w1053, lower limit=0.0) -> (In Range?=w1052:bool)  [unwired: 1 out]
          n892 = case shown="False" w1052 {
            tunnel: w1052 -> [_ _]
            tunnel: w1054 -> [w1058 _]
            tunnel: [w1057 w1066] -> w1051
            tunnel: w1053 -> [w1056 w1066]
            frame False {
              n893 = Greater?(x=w1058, y=w1056) -> (0:w1059:bool)
              n894 = case shown="True" w1059 {
                tunnel: w1058 -> [w1061 w1063]
                tunnel: [w1060 w1064] -> w1057
                frame False {
                  n895 = Add(x=w1061, y=100.0) -> (x+y=w1060:dbl)
                }
                frame True {
                  n896 = Subtract(x=w1063, y=100.0) -> (x-y=w1064:dbl)
                }
              }
            }
            frame True {
            }
          }
        }
        n897 = call "RDG822 Standard Waveform.vi"("Configure"=w999, "Amplitude (0.1 Vpp)"=w1002, "Frequency (1000 Hz)"=w1005, "DC Offset (0.00 V)"=w1003, "Output Channel (1: Channel 1)"=w1025, "Amplitude Unit (0: Vpp)"=w1007, "Phase (0 Degree)"=w1006, "error in (no error)"=w1027, "Duty Cycle (50 %)"=w1000) -> ("resulting string"=w1008:string, "error out"=w1024:errorcluster)  [unwired: 5 in]
        n898 = call "HTTPGetRequest_Inst.vi"("Send/Read/Download/Remove"=w1022, "error in (no error)"=w1024, "userdata="=w1008, "userID"=w1026) -> ("error out"=w1014:errorcluster, "ReqNum"=w1012:string)  [unwired: 5 in, 1 out]
        n899 = Build Path(base path=w1015, name or relative path=path "Results") -> (appended path=w1017:path)
        n900 = call "QueryDoneFlag.vi"("error in (no error)"=w1014, "ReqNum"=w1012) -> ("error out"=w1013:errorcluster)  [unwired: 9 in]
        n901 = call "HTTPGetRequest_Inst.vi"("Send/Read/Download/Remove"=w1021, "Path to FP"=w1017, "error in (no error)"=w1013, "ReqNum"=w1012) -> ("error out"=w1028:errorcluster)  [unwired: 5 in, 2 out]
        n902 = call "UnZipFile.vi"("error in (no error)"=w1028, "Zip name"=w1012, "Path to FP"=w1017) -> ("error out"=w1023:errorcluster, "File path"=w1019:path)  [unwired: 7 in]
        n903 = case shown="True" "RemoveReq?" {
          tunnel: w1023 -> [w1067 w1071]
          tunnel: [w1067 w1070] -> w1009
          tunnel: w1012 -> [_ w1068]
          frame False {
          }
          frame True {
            w1069 = u16 3 items=["Send", "Read", "Download", "Remove"] ("Send/Read/Download/Remove")
            n904 = call "HTTPGetRequest_Inst.vi"("Send/Read/Download/Remove"=w1069, "error in (no error)"=w1071, "ReqNum"=w1068) -> ("error out"=w1070:errorcluster)  [unwired: 6 in, 2 out]
          }
        }
        n905 = property on="Freq-Period" class="Str"(error in=w1009, "Visible"=w1010) -> (error out=w1035:errorcluster)  [unwired: 1 in, 1 out]
        n906 = property on="Freq/Period" class="Bool (strict)"(error in=w1009, "Visible"=w1010) -> (error out=w1031:errorcluster)  [unwired: 1 in, 1 out]
        n907 = property on="Ampl/HighL" class="Bool (strict)"(error in=w1031, "Visible"=w1010) -> (error out=w1030:errorcluster)  [unwired: 1 in, 1 out]
        n908 = property on="Ampl-HighL" class="Str"(error in=w1035, "Visible"=w1010) -> (error out=w1034:errorcluster)  [unwired: 1 in, 1 out]
        n909 = call "RDG822 Update Screen.vi"("error in"=w1009, "Path to file"=w1019) -> ("error out"=w1029:errorcluster, "Screen"=w1020:picture)  [unwired: 8 in]
        n910 = property on="Offset/LowL" class="Bool (strict)"(error in=w1030, "Visible"=w1010) -> (error out=w1011:errorcluster)  [unwired: 1 in, 1 out]
        n911 = property on="Offset-LowL" class="Str"(error in=w1034, "Visible"=w1010) -> (error out=w1033:errorcluster)  [unwired: 1 in, 1 out]
        n912 = local write "error out"(w1029) -> ()
        n913 = local write "Screen"(w1020) -> ()
        n914 = property on="Slider" class="Bool (strict)"(error in=w1011, "Visible"=w1010) -> ()  [unwired: 1 in, 2 out]
        n915 = property on="PhaseStr" class="Str"(error in=w1033, "Visible"=w1010) -> ()  [unwired: 1 in, 2 out]
        n916 = call "Time Delay5"() -> ("error out"=w1037:errorcluster)  [unwired: 11 in]
        n917 = property on="Out1" class="Bool (strict)"(error in=w1037, "Value"=FALSE ("Out1")) -> ()  [unwired: 1 in, 2 out]
      }
      event "Out2": Value Change {
        (unwired) 2 items=["Channel 1"=1, "Channel 2"=2] ("Output Channel (1: Channel 1)")
        # "Same as Out1 eventually"
        n918 = event-data() -> ()  [unwired: 1 in, 6 out]
      }
    }
  }
